vi "find.vi"() -> ()   [LabVIEW 2009]
uses:
  newCore/Variables/GlobalConAxisPI.vi
  newCore/Camera/lib/System Files/user.lib/atmcd32d.llb/Shutter_type typedef.ctl
  newCore/Camera/lib/System Files/user.lib/atmcd32d.llb/Shutter_mode typedef.ctl
  newCore/Camera/vi/GlobalSetGetConfigureCamera.vi
  newCore/Camera/vi/ccdChipPixels.vi
  <vilib>/vision/Image Controls.llb/IMAQ Rounding Mode.ctl
  newCore/Variables/patternImg.vi
  <vilib>/vision/Pattern Matching.llb/IMAQ Match Range Setting.ctl
  <vilib>/vision/Pattern Matching.llb/IMAQ Curve Parameters.ctl
panel:
  in  "Tab Control":T1(tab)
  out "Histogram":i32[][](graph)
  out "Trace":i32[][](graph)
  out "Point":dbl[][](graph)
  out "Image Out":T2(plugin-control)
  out "Image Number":u32
  out "acquired FPS":dbl
  out "Image":i32[][](graph)
  out "AM image":T2(plugin-control)
  out "Number of Particles":i32
  out "Image 2":dbl[][](graph)
  out "concatenated string":string
  out "Task":T3(ring)
  in  "PI SystemNumber":i32
  in  "WS File Tree":string(tree)
  out "Active pt3":path
  out "Workspace":path
  out "Stop Measurement":bool
  out "Buffer Overrun":bool
  out "Running":bool
  out "Global Stop":bool
  out "x-position":dbl format="%.3f"
  out "y-position":dbl format="%.3f"
  out "z-position":dbl format="%.3f"
  out "Auto Meas Progress":i32(slide) caption="Point 34 / 34"
  out "NxtAutMesPoint":i32
  out "Auto Measure Points":i32
  out "subarray":dbl[](array[numeric])
  out "Pattern":dbl[][](array[numeric])
  in  "Remove Outliers":i32
  in  "Filter":bool
  in  "Exclude / Include X":bool
  in  "X Start 2":dbl
  in  "X End 2":dbl
  in  "Y Start 2":dbl
  in  "Y End 2":dbl
  in  "Exclude / Include Y":bool
  in  "Measurement Parameter 1":T4 items=["Center of Mass X", "Center of Mass Y", "First Pixel X", "First Pixel Y", "Bounding Rect Left", "Bounding Rect Top", "Bounding Rect Right", "Bounding Rect Bottom", "Max Feret Diameter Start X", "Max Feret Diameter Start Y", "Max Feret Diameter End X", "Max Feret Diameter End Y", "Max Horiz. Segment Length Left", "Max Horiz. Segment Length Right", "Max Horiz. Segment Length Row", "-", "Bounding Rect Width", "Bounding Rect Height", "Bounding Rect Diagonal", "Perimeter", "Convex Hull Perimeter", "Holes' Perimeter", "Max Feret Diameter", "Equivalent Ellipse Major Axis", "Equivalent Ellipse Minor Axis", "Equivalent Ellipse Minor Axis (Feret)", "Equivalent Rect Long Side", "Equivalent Rect Short Side", "Equivalent Rect Diagonal", "Equivalent Rect Short Side (Feret)", "Average Horiz. Segment Length", "Average Vert. Segment Length", "Hydraulic Radius", "Waddel Disk Diameter", "-", "Area", "Holes' Area", "Particle & Holes' Area", "Convex Hull Area", "Image Area", "-", "Number of Holes", "Number of Horiz. Segments", "Number of Vert. Segments", "-", "Orientation", "Max Feret Diameter Orientation", "-", "% Area/Image Area", "% Area/(Particle & Holes' Area)", "Ratio of Equivalent Ellipse Axes", "Ratio of Equivalent Rect Sides", "-", "Elongation Factor", "Compactness Factor", "Heywood Circularity Factor", "Type Factor", "-", "Sum X", "Sum Y", "Sum XX", "Sum XY", "Sum YY", "Sum XXX", "Sum XXY", "Sum XYY", "Sum YYY", "-", "Moment of Inertia XX", "Moment of Inertia XY", "Moment of Inertia YY", "Moment of Inertia XXX", "Moment of Inertia XXY", "Moment of Inertia XYY", "Moment of Inertia YYY", "Norm. Moment of Inertia XX", "Norm. Moment of Inertia XY", "Norm. Moment of Inertia YY", "Norm. Moment of Inertia XXX", "Norm. Moment of Inertia XXY", "Norm. Moment of Inertia XYY", "Norm. Moment of Inertia YYY", "Hu Moment 1", "Hu Moment 2", "Hu Moment 3", "Hu Moment 4", "Hu Moment 5", "Hu Moment 6", "Hu Moment 7"]
  in  "Range Lower Value Par 1":dbl
  in  "Range Upper Value  Par 1":dbl
  in  "Ex/In Par 1":bool
  in  "Measurement Parameter 2":T4 items=["Center of Mass X", "Center of Mass Y", "First Pixel X", "First Pixel Y", "Bounding Rect Left", "Bounding Rect Top", "Bounding Rect Right", "Bounding Rect Bottom", "Max Feret Diameter Start X", "Max Feret Diameter Start Y", "Max Feret Diameter End X", "Max Feret Diameter End Y", "Max Horiz. Segment Length Left", "Max Horiz. Segment Length Right", "Max Horiz. Segment Length Row", "-", "Bounding Rect Width", "Bounding Rect Height", "Bounding Rect Diagonal", "Perimeter", "Convex Hull Perimeter", "Holes' Perimeter", "Max Feret Diameter", "Equivalent Ellipse Major Axis", "Equivalent Ellipse Minor Axis", "Equivalent Ellipse Minor Axis (Feret)", "Equivalent Rect Long Side", "Equivalent Rect Short Side", "Equivalent Rect Diagonal", "Equivalent Rect Short Side (Feret)", "Average Horiz. Segment Length", "Average Vert. Segment Length", "Hydraulic Radius", "Waddel Disk Diameter", "-", "Area", "Holes' Area", "Particle & Holes' Area", "Convex Hull Area", "Image Area", "-", "Number of Holes", "Number of Horiz. Segments", "Number of Vert. Segments", "-", "Orientation", "Max Feret Diameter Orientation", "-", "% Area/Image Area", "% Area/(Particle & Holes' Area)", "Ratio of Equivalent Ellipse Axes", "Ratio of Equivalent Rect Sides", "-", "Elongation Factor", "Compactness Factor", "Heywood Circularity Factor", "Type Factor", "-", "Sum X", "Sum Y", "Sum XX", "Sum XY", "Sum YY", "Sum XXX", "Sum XXY", "Sum XYY", "Sum YYY", "-", "Moment of Inertia XX", "Moment of Inertia XY", "Moment of Inertia YY", "Moment of Inertia XXX", "Moment of Inertia XXY", "Moment of Inertia XYY", "Moment of Inertia YYY", "Norm. Moment of Inertia XX", "Norm. Moment of Inertia XY", "Norm. Moment of Inertia YY", "Norm. Moment of Inertia XXX", "Norm. Moment of Inertia XXY", "Norm. Moment of Inertia XYY", "Norm. Moment of Inertia YYY", "Hu Moment 1", "Hu Moment 2", "Hu Moment 3", "Hu Moment 4", "Hu Moment 5", "Hu Moment 6", "Hu Moment 7"]
  in  "Range Lower Value Par 2":dbl
  in  "Range Upper Value Par 2":dbl
  in  "Ex/In Par 2":bool
  in  "Settings (GeometricMatching)":T7 {"Curve Parameters"."Extraction Mode" items=["Normal", "Uniform Regions"]; "Curve Parameters"."Edge Filter Size" items=["Fine", "Normal", "Contour Tracing"]; "Curve Parameters"."Max Endpoint Gap" min=0; "Curve Parameters"."Col Search Step Size" min=1 max=255 step=1; "Curve Parameters"."Row Search Step Size" min=1 max=255 step=1; "Curve Parameters"."Min Length" min=0; "Curve Parameters"."Edge Threshold" min=1 max=350 step=1; "Range Settings"."Max" format="%.2f"; "Range Settings"."Min" format="%.2f"; "Range Settings"."Match Constraints" items=["Rotation Angle (degrees)", "Scale Factor (%)", "Occlusion (%)"]; "Adv. Geometric Match Options 2"."Setup Data Item" items=["Curve Extraction Mode", "Curve Edge Threshold", "Curve Edge Filter Size", "Min Curve Length", "Curve Row Search Step Size", "Curve Col Search Step Size", "Curve Max Endpoint Gap", "Extract Closed Curves", "Enable Subpixel Curve Extraction", "Enable Correlation Score", "Enable Subpixel Accuracy", "Subpixel Iterations", "Subpixel Tolerance", "Initial Match List Length", "Enable Target Template Curve Score", "Min Match Separation Distance", "Min Match Separation Angle", "Min Match Separation Scale", "Max Match Overlap", "Enable Coarse Result", "Enable Calibration Support", "Enable Contrast Reversal", "Search Strategy", "Refinement Match Factor", "Subpixel Match Factor"]}
  in  "Square/Hexa":bool
  in  "Connectivity 4/8":bool
  in  "Manual":bool
  in  "Mode":enum16{"Gauss", "Radial", "Azimuthal"}(ring)
  in  "Focuswidth":dbl
  in  "Detection Modus":u16(ring) items=["Pattern", "Heuristic"]
  in  "NA":dbl
  in  "Measurement Time":i32 min=10 format="%.0d s"
  out "Counts":u32[](array[numeric])
  in  "Adjustment":bool
  in  "Autopoint-Autofocus Z":bool
  in  "Auto Measurement Time (ms)":i32 caption="Measurement Time (s)" min=10
  in  "Auto Defocussed Cam":bool
  in  "Point Defocussed Cam":bool
  in  "X-Position":dbl caption="X" min=0.0 max=200.0 step=0.1 format="%1.3f um"
  in  "Y-Position":dbl caption="Y" min=0.0 max=200.0 step=0.1 format="%1.3f um"
  in  "Z-Position":dbl caption="Z" min=0.0 max=200.0 step=0.1 format="%1.3f um"
  in  "Picture size":dbl min=0.1 max=200.0 format="%1.1f um"
  in  "Picture size 2":dbl min=0.1 max=200.0 format="%1.1f um"
  in  "Pixel time":dbl min=0.1 max=100.0 step=0.1 format="%.1f ms"
  in  "Resolution":dbl min=0.01 max=10.0 step=0.01 format="%.2f µm"
  in  "Laser  Profile":string
  in  "Save Files":bool
  in  "Axis":enum32{"x-y", "x-z", "y-x", "y-z", "z-x", "z-y"}(ring)
  out "Last Image File No":i32
  in  "CFD Settings":T8
  out "Measure. time":dbl format="%7.1f s"
  in  "Laser pulse duration":i32[](array[numeric]) min=2 max=100000 step=1 format="%d µs"
  # "Range"
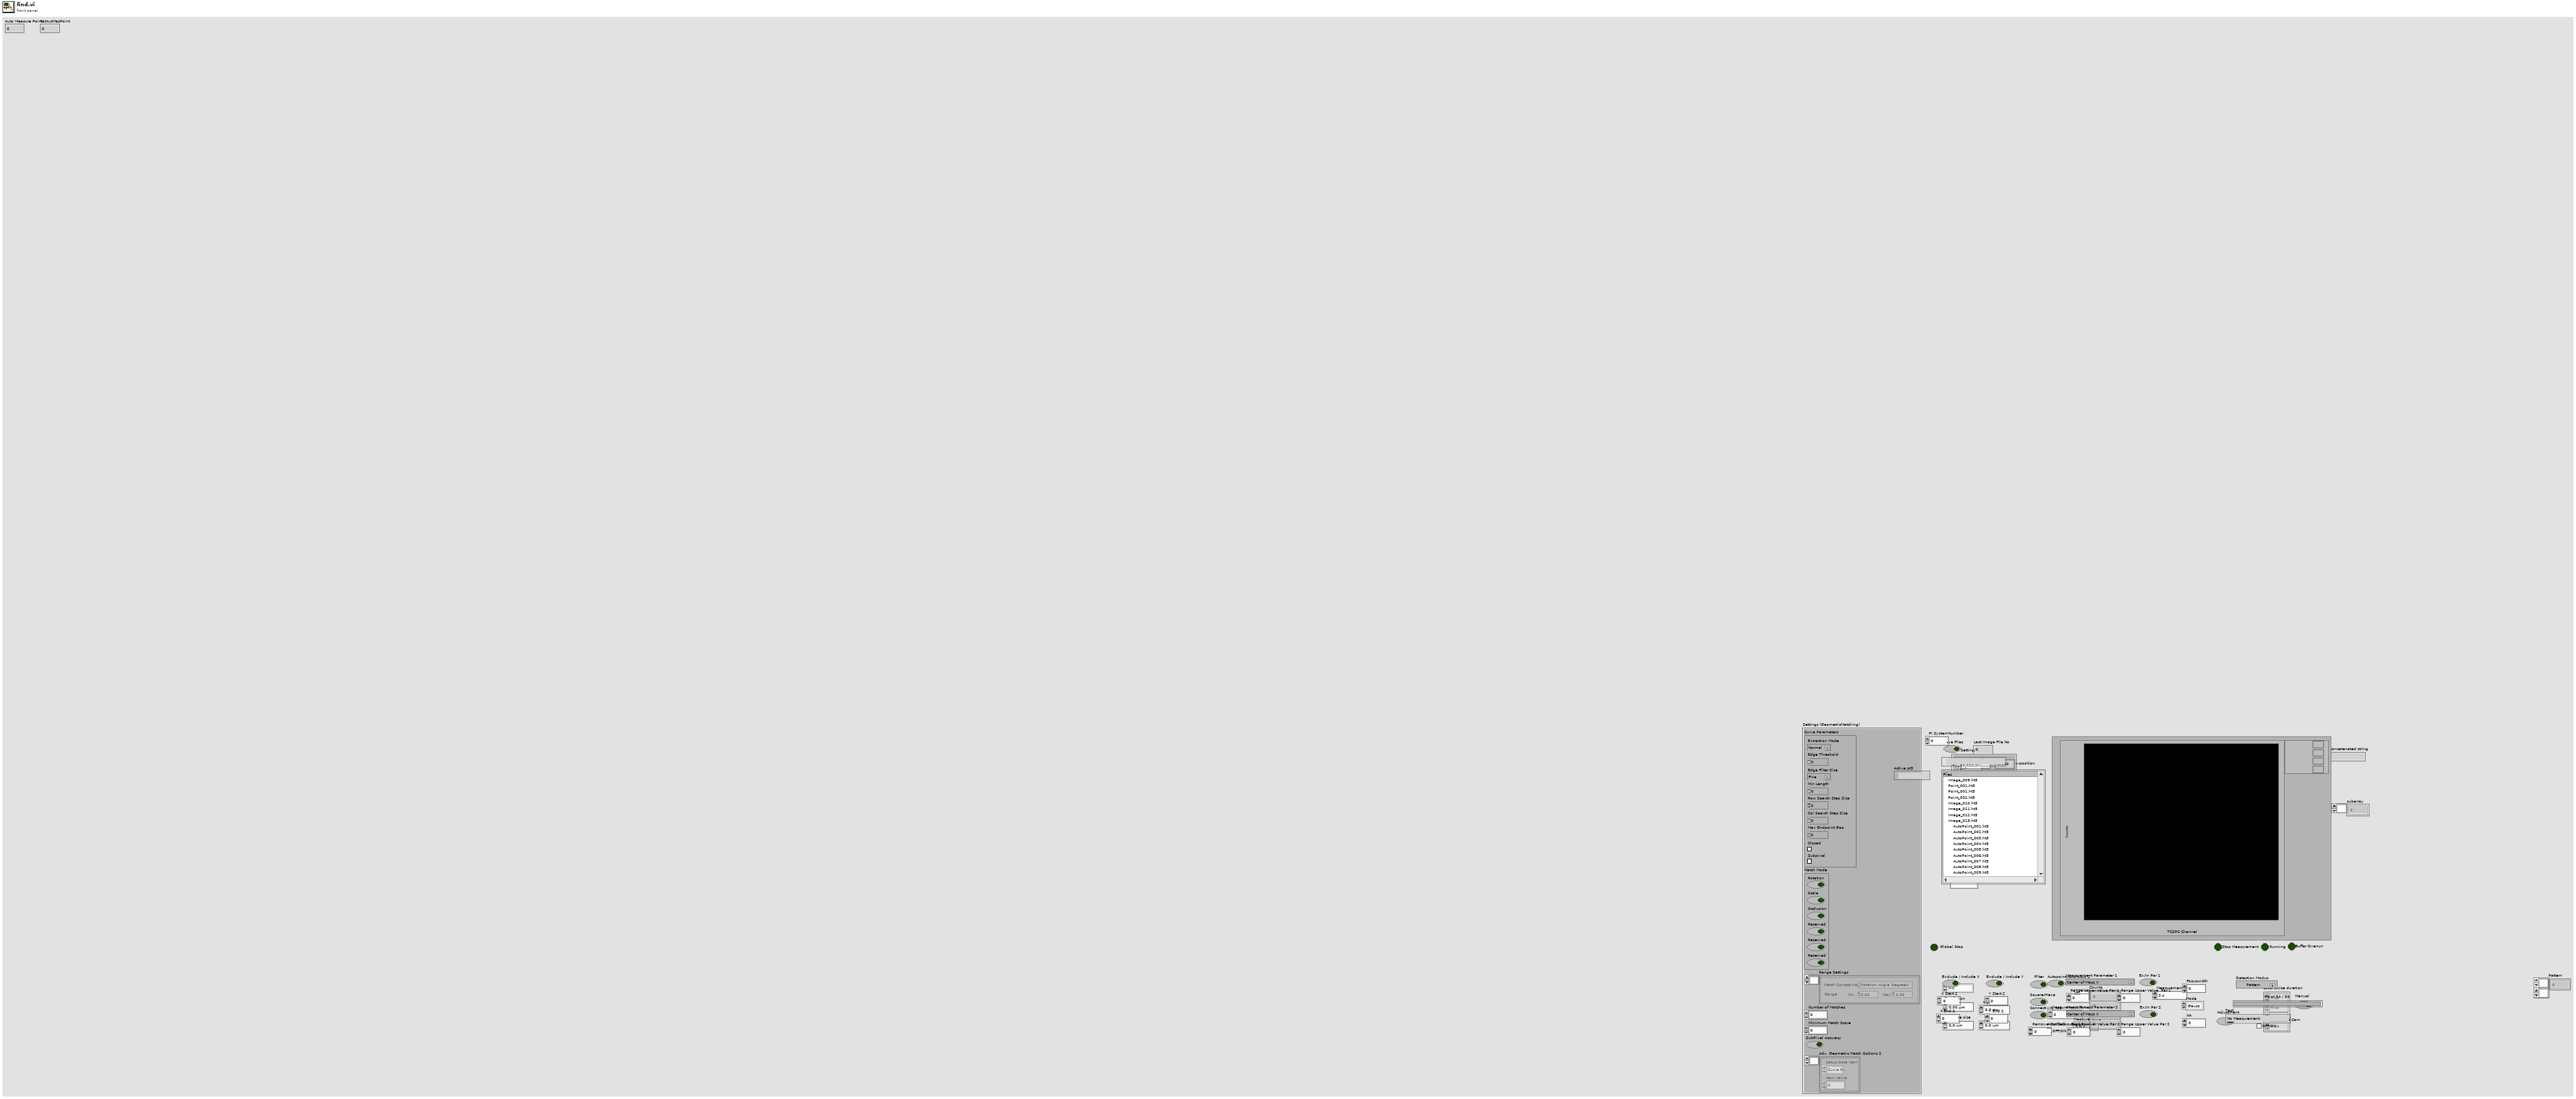
[diagram p1: front panel]
types:
  T1 = enum32{"TCSPC Histogram", "Trace", "CCD", "Backreflection", "Image", "AutoMesaurement"}
  T2 = typedef "IMAQ Image.ctl" = refnum<image>
  T3 = enum16{"No Measurement", "Aquire Image", "Point Measurement", "Multi Measurement", "Save Color Image", "Find Single Mol.", "Auto Measurement Control", "Auto Point", "Aquire Line Scan", "Grid Measurement", "Trapping", "Move Scanner"}
  T4 = typedef "Particle Parameters" = i32
  T5 = typedef "IMAQ Curve Parameters.ctl" = cluster{"Extraction Mode":u32, "Edge Threshold":i32, "Edge Filter Size":u32, "Min Length":i32, "Row Search Step Size":i32, "Col Search Step Size":i32, "Max Endpoint Gap":i32, "Closed":bool, "Subpixel":bool}
  T6 = typedef "IMAQ Match Range Setting.ctl" = cluster{"Match Constraints":u32, "Min":dbl, "Max":dbl}
  T7 = cluster{"Curve Parameters":T5, "Match Mode":cluster{"Rotation":bool, "Scale":bool, "Occlusion":bool, "Reserved":bool, "Reserved":bool, "Reserved":bool}, "Range Settings":T6[], "Number of Matches":i32, "Minimum Match Score":sgl, "SubPixel Accuracy":bool, "Adv. Geometric Match Options 2":cluster{"Setup Data Item":u16, "Item Value":dbl}[]}
  T8 = cluster{"Sync Level":i32, "Sync ZeroX":i32, "Sync Offset":i32, "Chan Settings":cluster{"CHx Level":i32, "CHx ZeroX":i32, "CHx Offset":i32}[]}
  T9 = enum16{"No Measurement", "Aquire Image", "Point Measurement", "Multi Measurement", "Save Color Image", "Find Single Mol.", "Auto Measurement Control", "Auto Point", "Aquire Line Scan", "Grid Measurement"}
  T10 = enum16{"none", "fast axis", "slow axis", "both axis", ""}
  T11 = enum16{"none", "fast axis", "slow axis", "both", ""}
  T12 = enum16{"target position", "relative position", "actual position", "position error"}
  T13 = enum16{"not a pt3 File", "Image File", "Point Measurement", "Auto Point"}
  T14 = enum16{"unknown", "pt3 File", "png Image", "bmp Image"}
  T15 = typedef "Shutter_mode typedef.ctl" = enum16{"Auto", "Open", "Close"}
  T16 = typedef "Shutter_type typedef.ctl" = enum16{"TTL Low", "TTL High"}
  T17 = enum16{"No Measurement", "Aquire Image", "Point Measurement", "Multi Measurement", "Save Color Image", "Find Single Mol.", "Auto Measurement Control", "Auto Point"}
  T18 = typedef "IMAQ Rounding Mode.ctl" = enum16{"Optimize", "Truncate"}
  T19 = cluster{"Measurement Parameter":T4, "Range Lower Value":dbl, "Range Upper Value":dbl, "Range":bool, "Measurement Type":bool}[]
  T20 = enum16{"not a pt3 File", "Image File", "Point Measurement", "Auto Point", "Line Scan"}
  T21 = cluster{"Comment":string, "Binning":i32, "Offset":i32, "AcquisitionTime (ms)":i32, "HardwareSerial":i32, "SyncDivider":i32, "Resolution (ps)":dbl, "CFD Settings":cluster{"Sync Level":i32, "Sync ZeroX":i32, "Sync Offset":i32, "Chan Settings":cluster{"CHx Level":i32, "CHx ZeroX":i32, "CHx Offset":i32}[]}, "ModuleInfo":cluster{"modelcode":i32, "versioncode":i32}[], "BaseResolution (ps)":dbl, "RefClockSource":i32, "ChanInfo":cluster{"CHx Level":i32, "CHx ZeroX":i32, "CHx Offset":i32, "CHx modidx":i32}[], "SyncRate":i32, "InputsEnabled":i64}
  T22 = cluster{"Dimensions":i32, "Time Per Pixel [ms]":dbl, "Acceleration":i32, "Pattern":i32, "X0":sgl, "Y0":sgl, "Z0":dbl, "PixX":i32, "PixY":i32, "PixResol":sgl, "TStartTo":sgl, "TStoptTo":sgl, "TStartFro":sgl, "TStopFro":sgl}
  T23 = cluster{"InpRateFilePos":i64, "StopAfterFilePos":i64}
  T24 = cluster{"X-Position":dbl, "Y-Position":dbl, "Z-Position":dbl}
  T25 = cluster{"File No":i32, "File Path":path, "Parent File":i32, "File Type":enum16{"unknown", "pt3 File", "png Image", "bmp Image"}, "Measurement Type":enum16{"not a pt3 File", "Image File", "Point Measurement", "Auto Point", "Line Scan", "Grid Scan"}, "Upper Left":cluster{"x-Position":dbl, "y-Position":dbl, "z-Position":dbl}, "Pixels":i32[], "Scan Axis":enum32{"x-y", "x-z", "y-z"}, "Resolution":dbl, "PixelTime":dbl}
  T26 = enum16{"not a pt3 File", "Image File", "Point Measurement", "Auto Point", "Line Scan", "Grid Scan"}
  T27 = cluster{"Ident":string, "Format Version":string, "Creator Name":string, "Creator Version":string, "File Time":string, "Comment":string, "Laser":i32, "Binning":i32, "Offset":i32, "AcquisitionTime (ms)":i32, "HardwareSerial":i32, "SyncDivider":i32, "Resolution (ps)":dbl, "Rates":dbl[], "SyncRate":dbl, "CFD Settings":cluster{"Sync Level":i32, "Sync ZeroX":i32, "Sync Offset":i32, "Chan Settings":cluster{"CHx Level":i32, "CHx ZeroX":i32, "CHx Offset":i32}[]}}
  T28 = cluster{"x-Position":dbl, "y-Position":dbl, "z-Position":dbl}
  T29 = typedef "Image Type" = u32
  T30 = cluster{"MesaurementSelection[0]":cluster{"Measurement Parameter":T4, "Range Lower Value":dbl, "Range Upper Value":dbl, "Range":bool, "Measurement Type":bool}, "MesaurementSelection[1]":cluster{"Measurement Parameter":T4, "Range Lower Value":dbl, "Range Upper Value":dbl, "Range":bool, "Measurement Type":bool}, "MesaurementSelection[2]":cluster{"Measurement Parameter":T4, "Range Lower Value":dbl, "Range Upper Value":dbl, "Range":bool, "Measurement Type":bool}, "MesaurementSelection[3]":cluster{"Measurement Parameter":T4, "Range Lower Value":dbl, "Range Upper Value":dbl, "Range":bool, "Measurement Type":bool}, "MesaurementSelection[4]":cluster{"Measurement Parameter":T4, "Range Lower Value":dbl, "Range Upper Value":dbl, "Range":bool, "Measurement Type":bool}, "MesaurementSelection[5]":cluster{"Measurement Parameter":T4, "Range Lower Value":dbl, "Range Upper Value":dbl, "Range":bool, "Measurement Type":bool}, "MesaurementSelection[6]":cluster{"Measurement Parameter":T4, "Range Lower Value":dbl, "Range Upper Value":dbl, "Range":bool, "Measurement Type":bool}, "MesaurementSelection[7]":cluster{"Measurement Parameter":T4, "Range Lower Value":dbl, "Range Upper Value":dbl, "Range":bool, "Measurement Type":bool}, "MesaurementSelection[8]":cluster{"Measurement Parameter":T4, "Range Lower Value":dbl, "Range Upper Value":dbl, "Range":bool, "Measurement Type":bool}}
  T31 = cluster{"Measurement Parameter":T4, "Range Lower Value":dbl, "Range Upper Value":dbl, "Range":bool, "Measurement Type":bool}
  T32 = typedef "IMAQ Point" = cluster{"X":sgl, "Y":sgl}
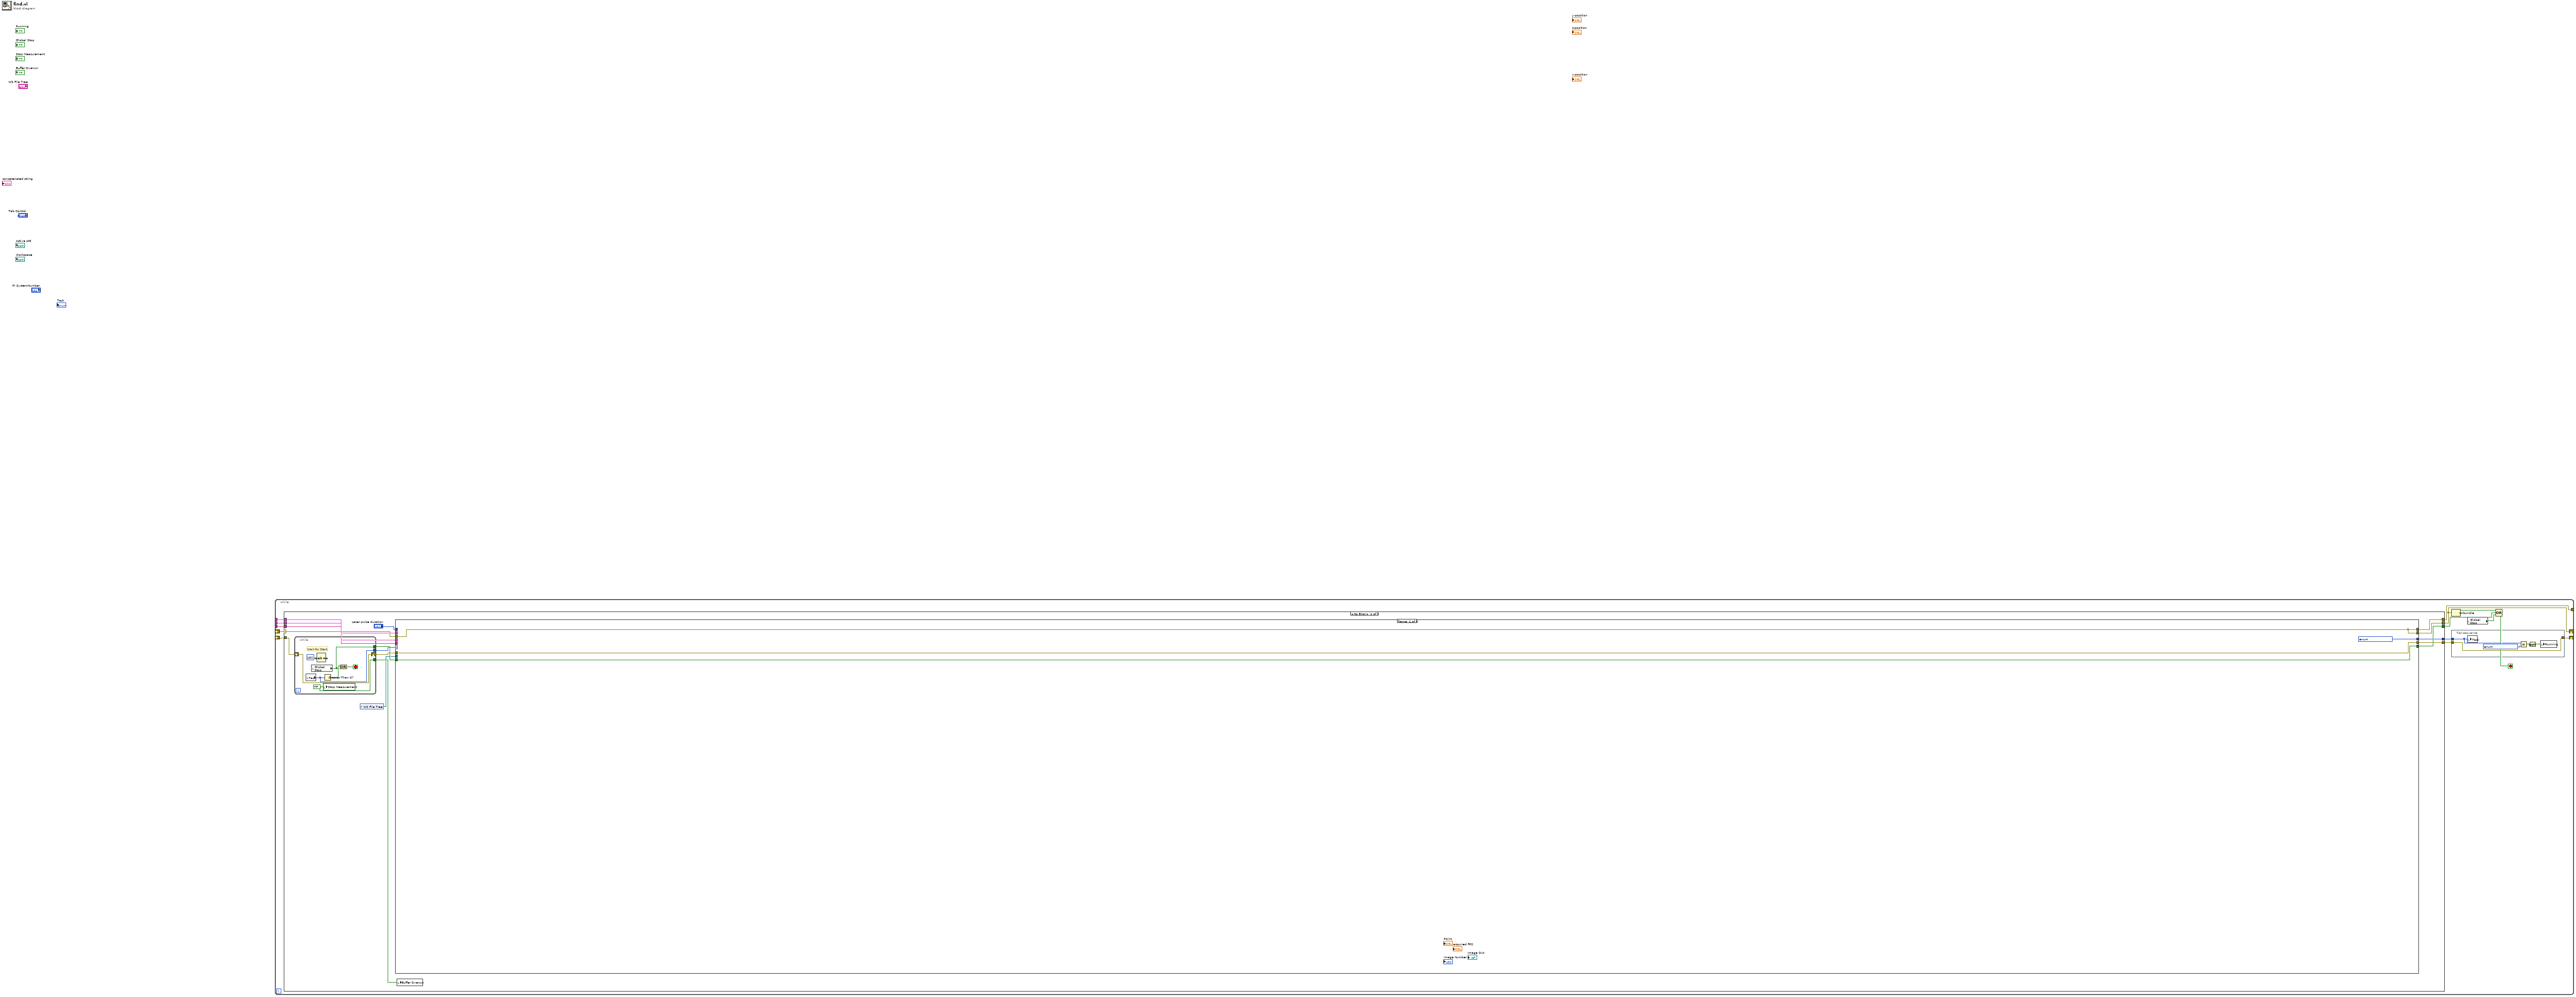
[diagram p0: block diagram]
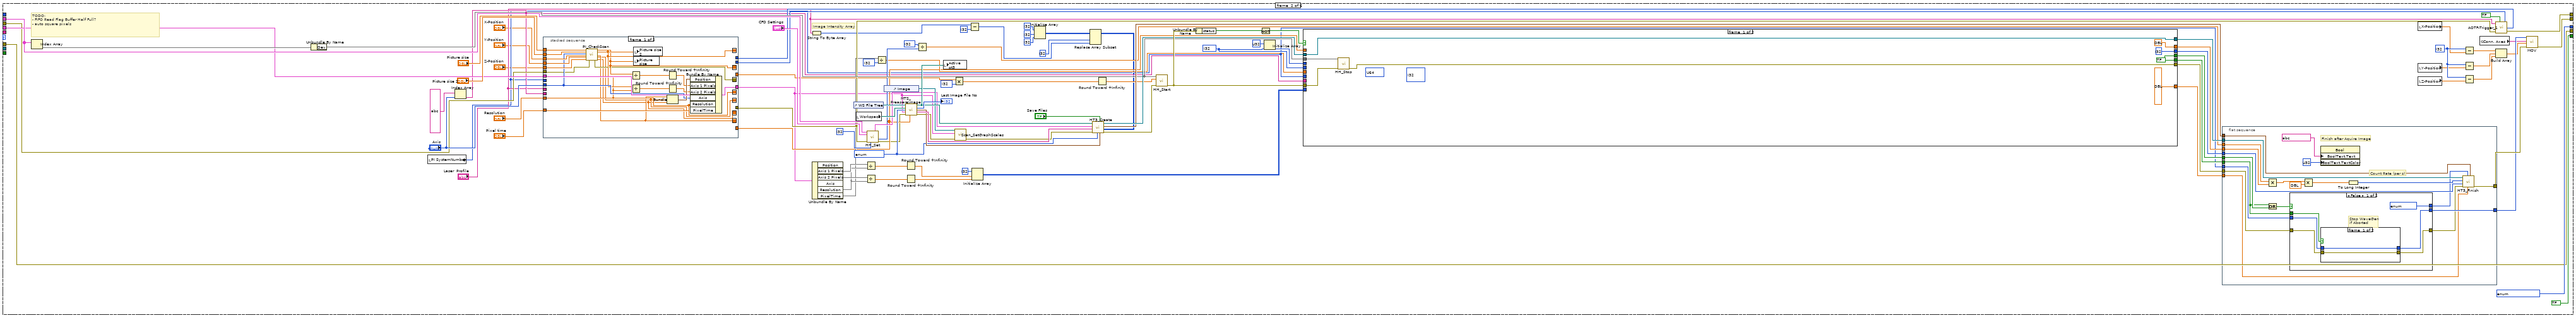
[diagram p2: hidden frame]
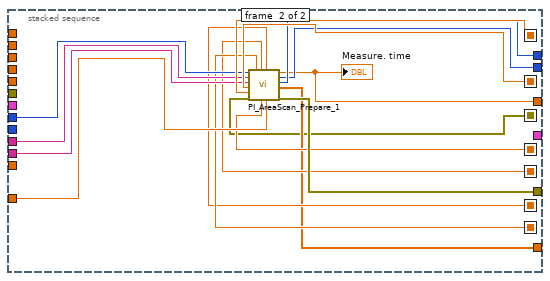
[diagram p3: hidden frame]
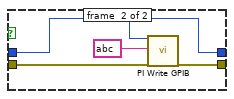
[diagram p4: hidden frame]
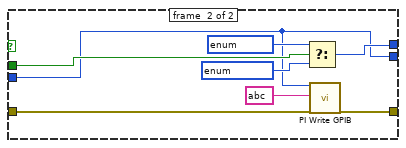
[diagram p5: hidden frame]
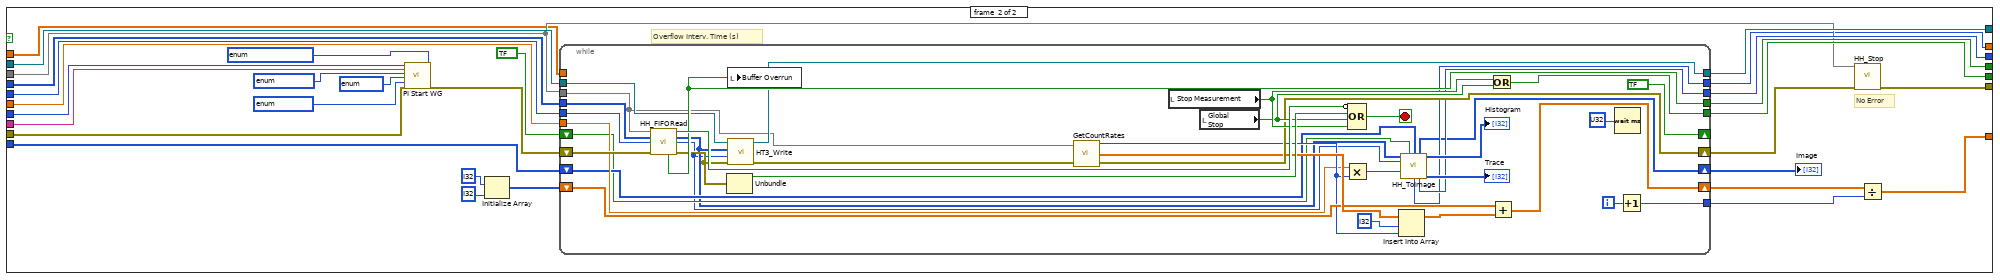
[diagram p6: hidden frame]
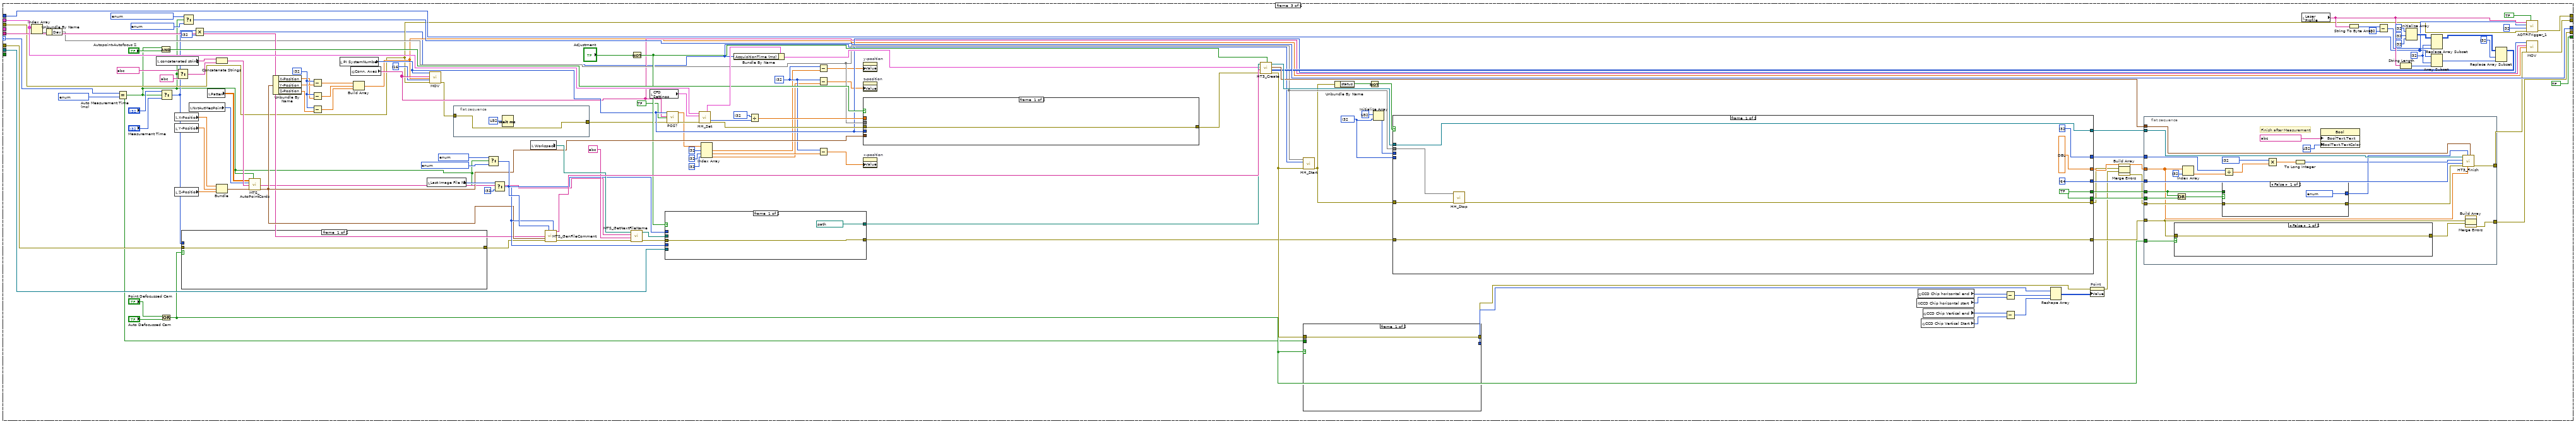
[diagram p7: hidden frame]
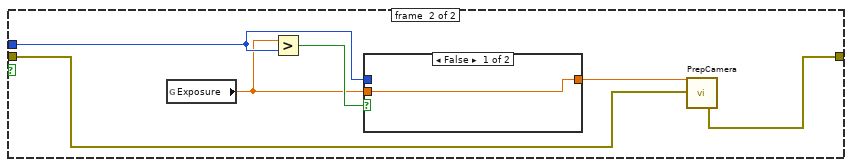
[diagram p8: hidden frame]
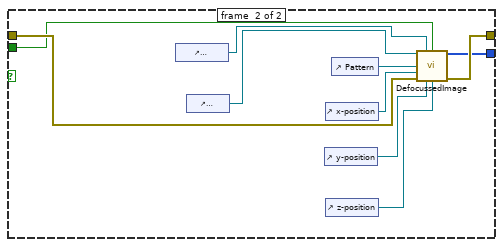
[diagram p10: hidden frame]
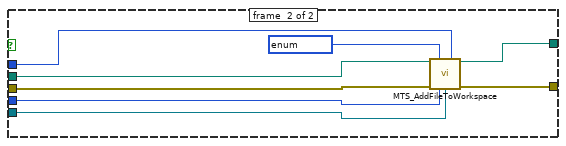
[diagram p11: hidden frame]
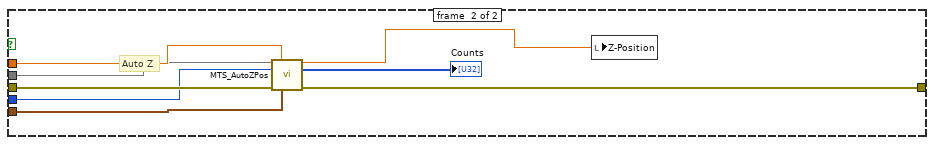
[diagram p12: hidden frame]
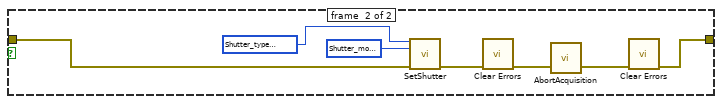
[diagram p13: hidden frame]
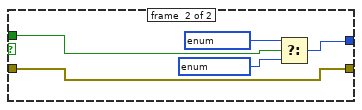
[diagram p14: hidden frame]
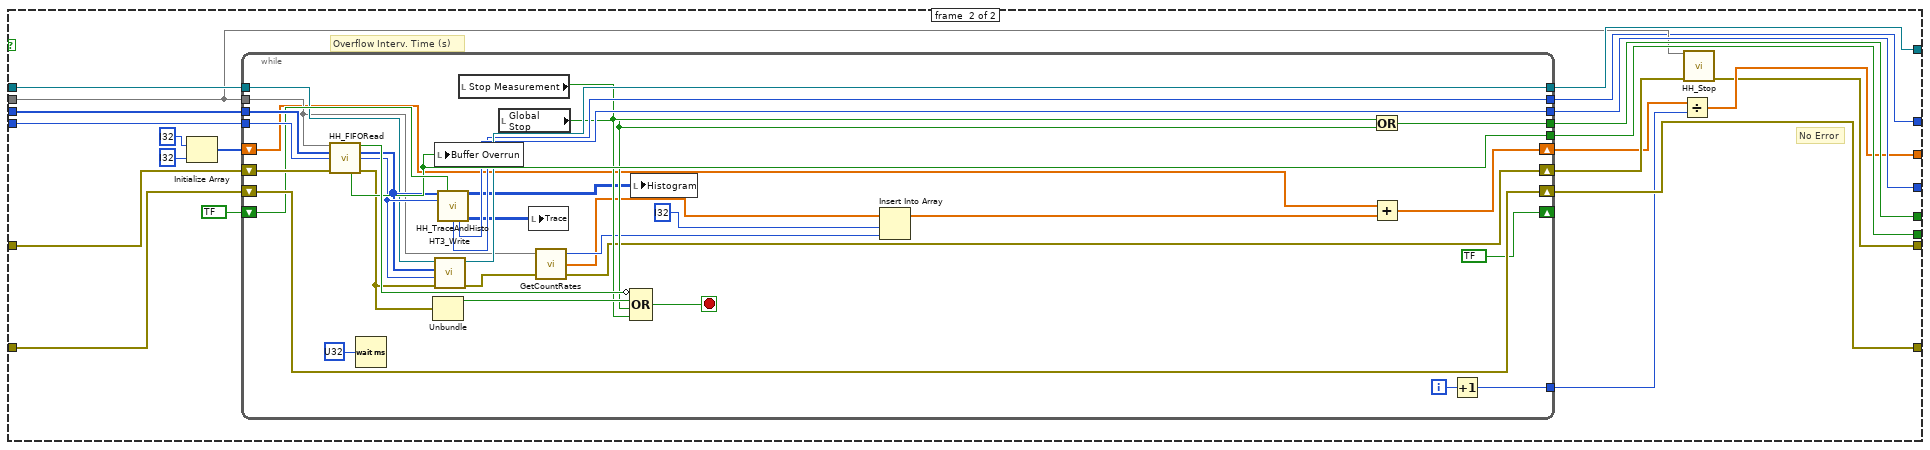
[diagram p15: hidden frame]
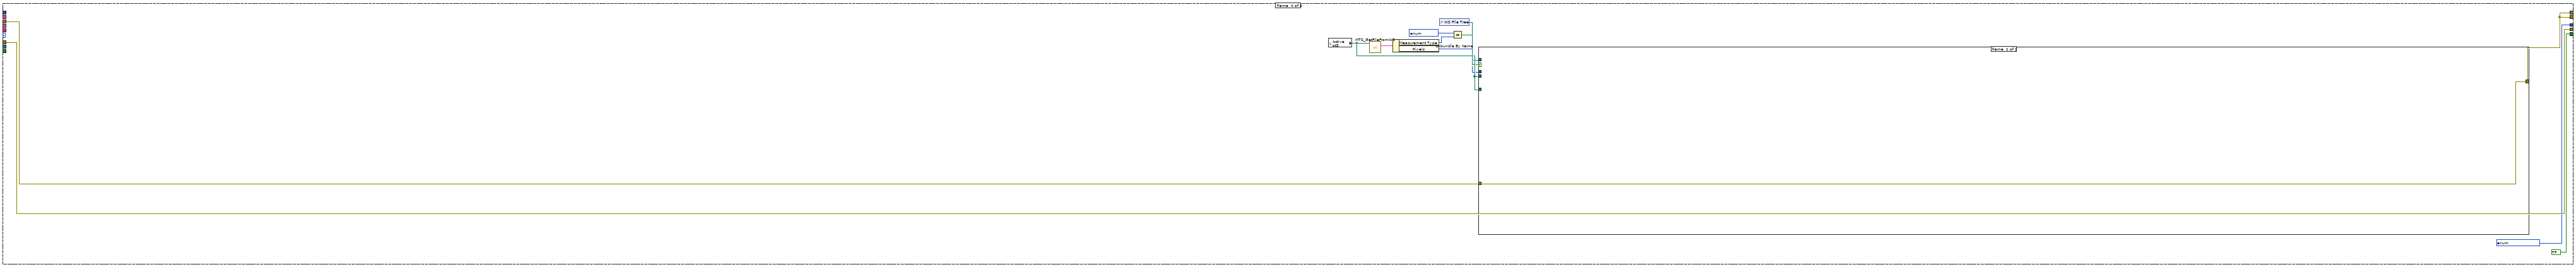
[diagram p16: hidden frame]
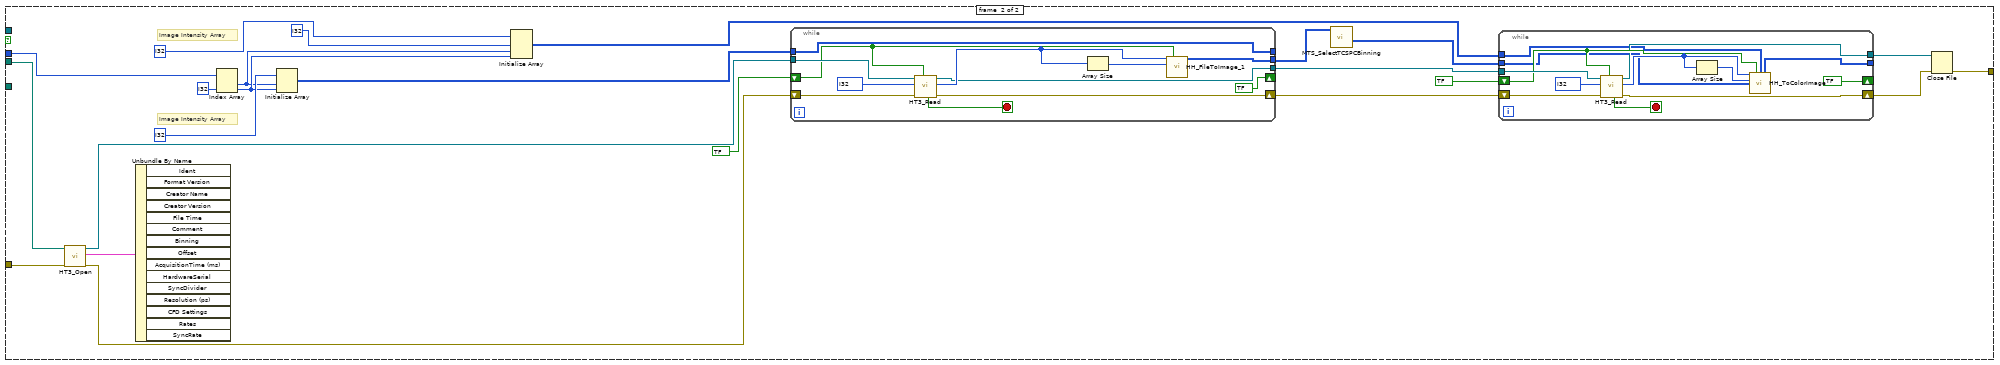
[diagram p17: hidden frame]
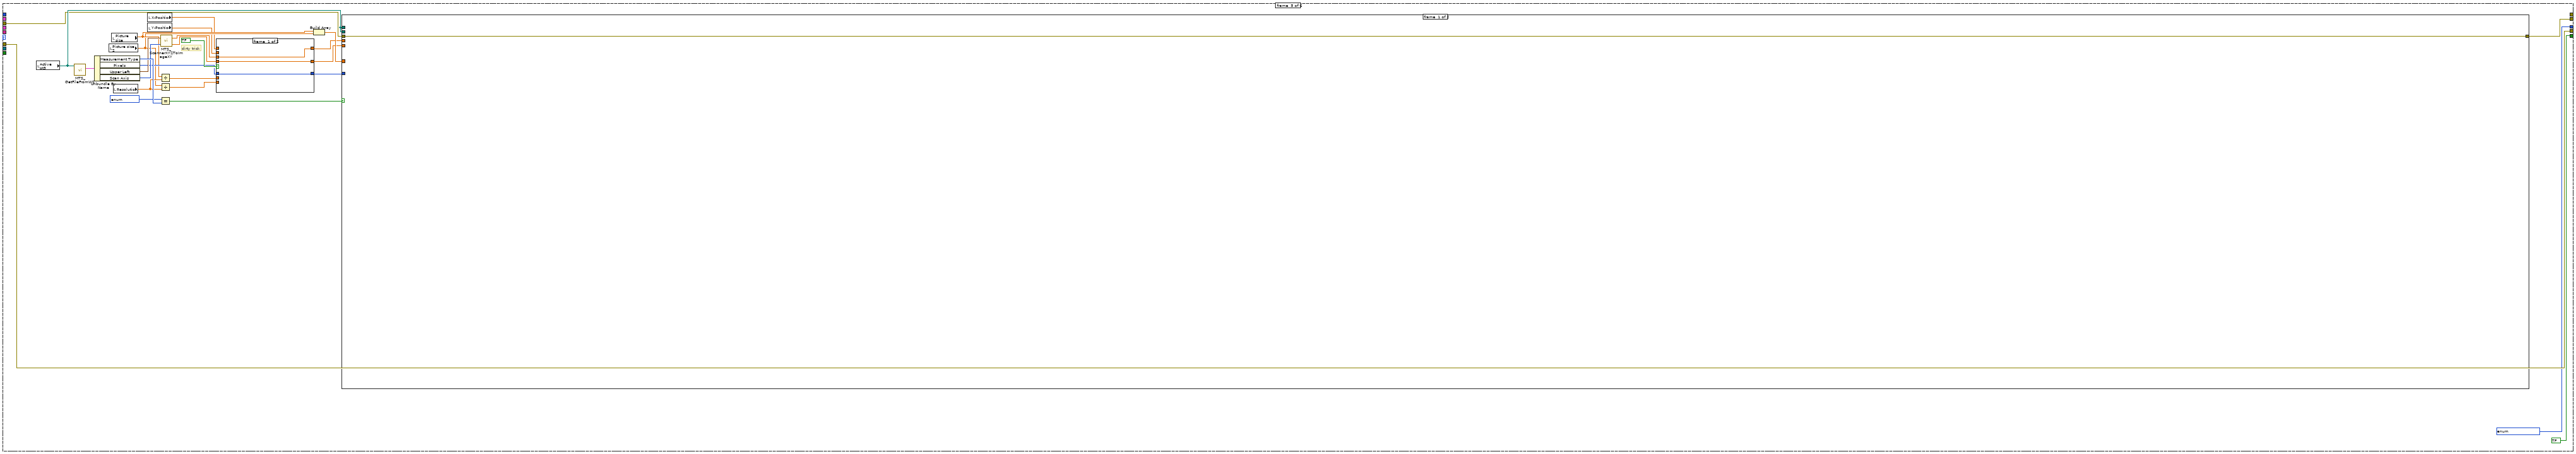
[diagram p18: hidden frame]
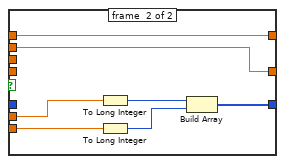
[diagram p19: hidden frame]
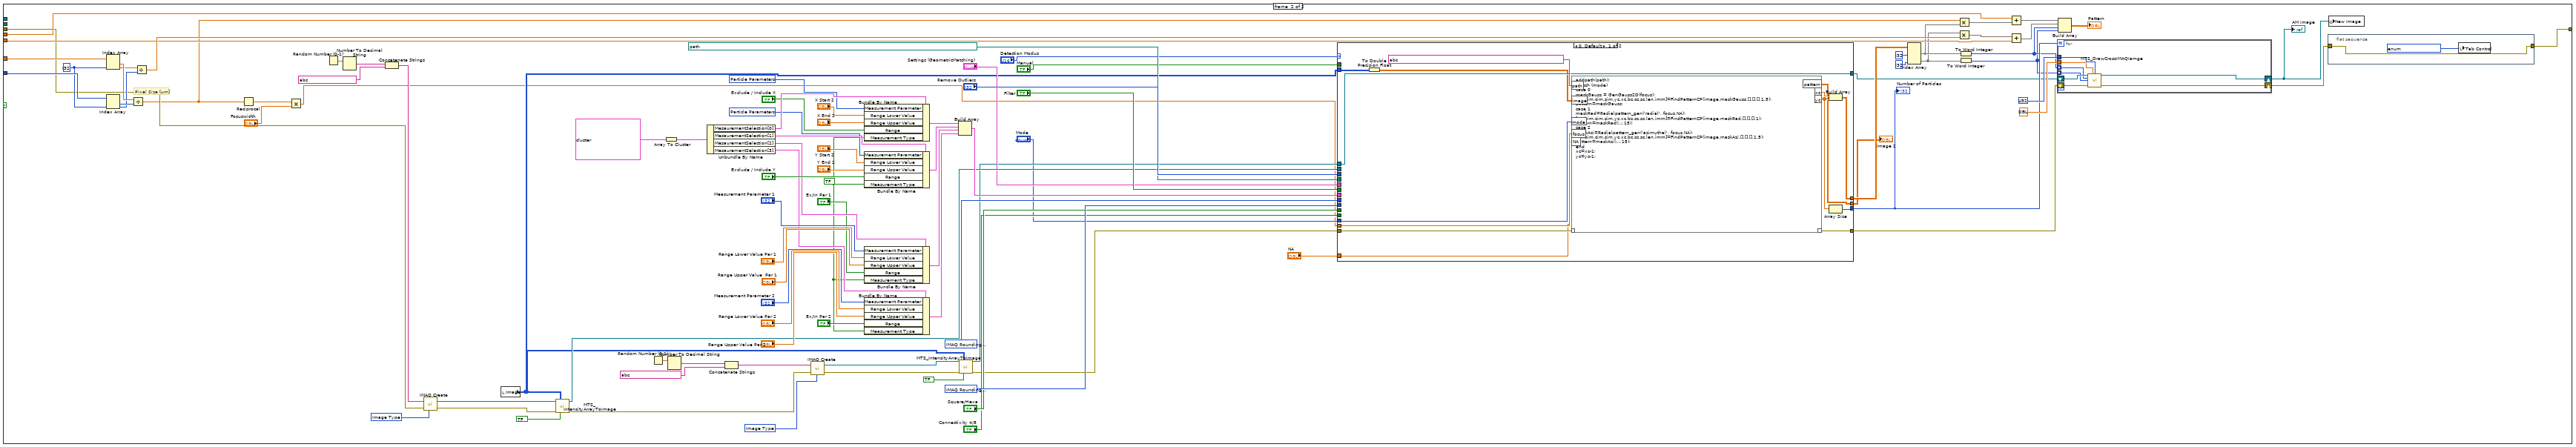
[diagram p20: hidden frame]
diagram:
  n1 = while {
    shift-right: [w7] -> _
    shift-left: _ -> [w4]
    shift-right: [w9] -> _
    shift-left: _ -> [w14]
    tunnel: _ -> [w8]
    tunnel: _ -> [w3]
    tunnel: [w2] -> _
    tunnel: _ -> [w1]
    stop <- w12 stop-if-true
    n2 = case shown="No Error" w4 {
      selector: w4 -> [w20 w892]
      tunnel: w14 -> [w30 w894]
      tunnel: [w29 bool ? ("Global Stop")] -> w11
      tunnel: [w25 w894] -> w10
      tunnel: w8 -> [w24 _]
      tunnel: [w23 w892] -> w7
      tunnel: [w21 T9 ? ("Do Measurement")] -> w5
      tunnel: w3 -> [w18 _]
      tunnel: [w17 w892] -> w2
      tunnel: w1 -> [w15 _]
      frame #0 {
        n3 = while {
          shift-right: [w890] -> w26
          shift-left: w30 -> [w890]
          tunnel: [w885] -> w28
          tunnel: [w887] -> w27
          tunnel: [w886] -> w22
          stop <- w891 stop-if-true
          w886 = bool ? ("FiFo Overrun")
          # "Wait for Start"
          n4 = local read "Task"() -> (w885:T3)
          n5 = local read "Global Stop"() -> (w887:bool)
          n6 = Wait (ms)(milliseconds to wait=u32 ?) -> ()  [unwired: 1 out]
          n7 = Greater Than 0?(x=w885) -> (x > 0?=w889:bool)
          n8 = local write "Stop Measurement"(w886) -> ()
          n9 = Or(x=w889, y=w887) -> (x .or. y?=w891:bool)
        }
        n10 = control-ref of="WS File Tree"() -> (w19:refnum<vi>)
        n11 = case shown="\"Find Single Mol.\"" w28 {
          selector: w28 -> [_ _ w397 _ _ _]
          tunnel: w20 -> [w31 w79 w305 w580 w649 w848]
          tunnel: [w31 w49 w353 w569 w647 w848] -> w23
          tunnel: [w32 bool ? ("Global Stop") bool ? ("Global Stop") bool ? ("Global Stop") bool ? ("Global Stop") bool ? ("Global Stop")] -> w29
          tunnel: w27 -> [w32 _ _ _ _ _]
          tunnel: w26 -> [w34 w63 w304 w579 w648 w849]
          tunnel: [w34 w63 w418 w579 w648 w847] -> w25
          tunnel: w24 -> [_ w129 w355 _ _ _]
          tunnel: [T9 ? ("Do Measurement") T9 ? ("Do Measurement") w396 T9 ? ("Do Measurement") T17 ? ("Do Measurement") w846] -> w21
          tunnel: w19 -> [_ _ w386 _ _ _]
          tunnel: w18 -> [_ w107 _ _ _ _]
          tunnel: [w31 w81 w379 w569 _ _] -> w17
          tunnel: "Laser pulse duration" -> [_ _ w361 _ _ _]
          tunnel: w15 -> [_ _ w352 _ _ _]
          frame #0 {
          }
          frame #1 {
            w42 = i32 ?
            w73 = T20 ? ("Measurement Type")
            w110 = i32 ? ("dimension size")
            # "TODO:\n- FIFO Read Flag Buffer Half Full?\n- auto square pixels"
            # "Image Intensity Array"
            n12 = Index Array(array=w129) -> (element=w128)  [unwired: 1 in]
            n13 = Unbundle By Name(w128) -> ("Dev"=w101)
            n14 = local read "PI SystemNumber"() -> (w51:i32)
            n15 = Index Array(array=string[] ? ("Array"), index="Axis") -> (element=w56:string)
            n16 = stacked-sequence {
              seq-local: [w141 _] -> [_ w168]
              seq-local: [w140 _] -> [_ w169]
              seq-local: [w139 _] -> [_ w164]
              seq-local: [w135 _] -> [_ w162]
              seq-local: [w134 _] -> [_ w161]
              seq-local: [w133 _] -> [_ w160]
              seq-local: [w136 _] -> [_ w156]
              tunnel: "Picture size" -> [w154 _]
              tunnel: "Picture size 2" -> [w153 _]
              tunnel: w107 -> [w152 _]
              tunnel: "X-Position" -> [w151 _]
              tunnel: "Y-Position" -> [w150 _]
              tunnel: "Z-Position" -> [w149 _]
              tunnel: "Axis" -> [w143 _]
              tunnel: "Resolution" -> [w139 _]
              tunnel: [w142 _] -> w35
              tunnel: [_ w170] -> w80
              tunnel: w79 -> [w137 _]
              tunnel: w56 -> [_ w167]
              tunnel: "Laser  Profile" -> [_ w166]
              tunnel: "Pixel time" -> [w138 w165]
              tunnel: w51 -> [_ w163]
              tunnel: [_ w155] -> w76
              tunnel: [_ w159] -> w75
              tunnel: [_ w158] -> w74
              tunnel: [_ w157] -> w66
              frame #0 {
                n17 = call "PI_CheckScan.vi"("Picture size"=w154, "Picture size 2"=w153, "Axis"=w143, "x-Position"=w151, "y-Position"=w150, "z-Position"=w149, "error in (no error)"=w137) -> ("error out"=w136:errorcluster, "Picture size out"=w140:dbl, "Picture size out 2"=w141:dbl, "a0"=w135:dbl, "b0"=w134:dbl, "c0"=w133:dbl)  [unwired: 7 in]
                n18 = Divide(x=w140, y=w139) -> (x/y=w146:dbl)
                n19 = Divide(x=w141, y=w139) -> (x/y=w147:dbl)
                n20 = local write "Picture size 2"(w141) -> ()
                n21 = local write "Picture size"(w140) -> ()
                n22 = Round Toward +Infinity(x=w146) -> (ceil(x): smallest int >= x=w145:dbl)
                n23 = Round Toward +Infinity(x=w147) -> (ceil(x): smallest int >= x=w144:dbl)
                n24 = Bundle("a0"=w135, "b0"=w134, "c0"=w133) -> (w148:cluster{"a0":dbl, "b0":dbl, "c0":dbl})  [unwired: 1 in]
                n25 = Bundle By Name(cluster=w152, "Position"=w148, "Axis 1 Pixels"=w145, "Axis 2 Pixels"=w144, "Axis"=w143, "Resolution"=w139, "PixelTime"=w138) -> (w142:cluster{})
              }
              frame #1 {
                n26 = call "PI_AreaScan_Prepare_1.vi"("System"=w163, "Laser"=w166, "Axis"=w167, "da"=w169, "db"=w168, "error in (no error)"=w156, "a0"=w162, "b0"=w161, "Resolution"=w164, "c0"=w160, "Pixel time"=w165) -> ("Tacq"=w155:dbl, "lp"=w158:i32, "ap"=w159:i32, "Trigger"=w157:dbl[], "error out"=w170:errorcluster)  [unwired: 4 in]
                "Measure. time" <- w155
              }
            }
            n27 = String To Byte Array(string="Laser  Profile") -> (unsigned byte array=w58:u8[])
            n28 = Unbundle By Name(w35) -> ("Axis 1 Pixels"=w88, "Axis 2 Pixels"=w89, "Resolution"=w86, "PixelTime"=w70)  [unwired: 2 out]
            n29 = control-ref of="WS File Tree"() -> (w113:refnum<vi>)
            n30 = local read "Workspace"() -> (w118:path)
            n31 = Divide(x=w88, y=w86) -> (x/y=w97:dbl)
            n32 = Divide(x=w89, y=w86) -> (x/y=w99:dbl)
            n33 = call "HH_Set.vi"("Device List"=w129, "CFD Settings"="CFD Settings", "error in (no error)"=w80, "SyncDiv"=i32 ?) -> ("ht3 header out"=w93:T21, "Sync Rate"=w91:i32, "error out"=w65:errorcluster)  [unwired: 7 in, 2 out]
            n34 = Divide(x=w70, y=i32 ?) -> (x/y=w68:dbl)
            n35 = control-ref of="Image"() -> (w95:refnum<vi>)
            n36 = Round Toward +Infinity(x=w97) -> (ceil(x): smallest int >= x=w96:dbl)
            n37 = Round Toward +Infinity(x=w99) -> (ceil(x): smallest int >= x=w98:dbl)
            n38 = call "MTS_PreapareImage.vi"("WS File Tree"=w113, "Workspace"=w118, "Measurement Type"=w73, "Image Measurent Parameters"=w35, "error in"=w65, "Trigger"=w66) -> ("File Name (dup)"=w103:path, "File No"=→"Last Image File No":i32, "Image Header"=w105:T22, "Comment"=w106:string, "error out"=w64:errorcluster)  [unwired: 5 in]
            n39 = Divide(x=i32 ?, y=w91) -> (x/y=w72:dbl)
            n40 = local write "Active pt3"(w103) -> ()
            n41 = Multiply(x=w76, y=i32 ?) -> (x*y=w85:dbl)
            n42 = call "Scan_SetGraphScales.vi"("error in (no error)"=w64, "Image Measurent Parameters"=w35, "Image"=w95) -> ("error out"=w94:errorcluster)  [unwired: 8 in]
            n43 = Subtract(x=w58, y=i32 ?) -> (x-y=w57:i32[])
            n44 = Initialize Array(i32 ? ("element"), w96, w98) -> (w69:i32[][])
            n45 = Initialize Array(i32 ?, i32 ?, i32 ?) -> (w55:i32[][])
            n46 = Replace Array Subset(array=w55, new element=w57, index (col)=i32 ?) -> (w53:i32[][])  [unwired: 1 in]
            n47 = call "HT3_Create.vi"("Laser"=w53, "Image Header in"=w105, "Save pt3"="Save Files", "Measurement Type"=w73, "error in"=w94, "Comment"=w106, "ht3 Header in"=w93, "File Path"=w103) -> ("error out"=w119:errorcluster, "FileHeaderPos"=w109:T23, "refnum out"=w117:refnum<file>)  [unwired: 1 in]
            n48 = Round Toward +Infinity(x=w85) -> (ceil(x): smallest int >= x=w83:dbl)
            n49 = call "HH_Start.vi"("Device Index"=w101, "Acq. Time"=w83, "error in (no error)"=w119) -> ("error out"=w126:errorcluster)  [unwired: 11 in, 1 out]
            n50 = Unbundle By Name(w126) -> ("status"=w127:bool)
            n51 = Not(x=w127) -> (.not. x?=w125:bool)
            n52 = Initialize Array(u32 ?, w110) -> (w122:u32[])
            n53 = case shown="True" w125 {
              tunnel: [w218 w249] -> w124
              tunnel: w51 -> [_ w244]
              tunnel: w126 -> [w219 w245]
              tunnel: w101 -> [w217 w236]
              tunnel: w69 -> [_ w221]
              tunnel: w122 -> [_ w243]
              tunnel: w110 -> [_ w242]
              tunnel: [w216 w241] -> w121
              tunnel: [w216 w240] -> w120
              tunnel: w117 -> [w215 w239]
              tunnel: [w215 w238] -> w116
              tunnel: [i32 ? ("Num Records Total") w237] -> w115
              tunnel: [dbl ? w230] -> w114
              tunnel: w56 -> [_ w233]
              tunnel: [dbl[] ? w227] -> w71
              tunnel: w68 -> [_ w223]
              tunnel: w66 -> [_ w222]
              frame #0 {
                (unwired) i32[][] ? ("Image Array Out")
                (unwired) u64[] ? ("Histograms")
                w216 = bool ? ("Stop Measurement")
                n54 = call "HH_Stop.vi"("Device Index"=w217, "error in (no error)"=w219) -> ("error out"=w218:errorcluster)  [unwired: 12 in, 1 out]
              }
              frame #1 {
                # "Overflow Interv. Time (s)"
                # "No Error"
                n55 = call "PI Start WG.vi"("System no."=w244, "axis"=w233, "Generator"=T10 ?, "Init DDL"=T11 ?, "increment"=T11 ?, "error in"=w245, "saved data"=T12 ?) -> ("error out"=w246:errorcluster)  [unwired: 12 in]
                n56 = Initialize Array(i32 ?, i32 ?) -> (w224:i32[])
                n57 = while {
                  tunnel: w236 -> [w269]
                  tunnel: w243 -> [w285]
                  tunnel: w242 -> [w284]
                  shift-right: [w270] -> w248
                  shift-left: w246 -> [w286]
                  shift-right: [bool ? ("Reset")] -> _
                  shift-left: bool ? ("Reset") -> [w257]
                  tunnel: [w278] -> w241
                  tunnel: [w274] -> w240
                  tunnel: w239 -> [w276]
                  tunnel: [w275] -> w238
                  tunnel: [w253] -> w237
                  tunnel: [w252] -> w230
                  shift-right: [w266] -> w229
                  shift-left: w224 -> [w264]
                  tunnel: [w263] -> w228
                  tunnel: w223 -> [w260]
                  tunnel: w222 -> [_]
                  shift-right: [w251] -> w220
                  shift-left: w221 -> [w259]
                  i -> [w262]
                  stop <- w283 stop-if-true
                  n58 = call "HH_FIFORead.vi"("Device Index"=w269, "Buffer In"=w285, "Count"=w284, "error in (no error)"=w286) -> ("OK"=w279:bool, "Buffer Out"=w256:u32[], "Data Count"=w255:i32, "FiFo Overrun"=w278:bool, "error out"=w277:errorcluster)  [unwired: 7 in]
                  n59 = Unbundle(w277) -> ("status"=w282:bool)  [unwired: 2 out]
                  n60 = local write "Buffer Overrun"(w278) -> ()
                  n61 = call "HT3_Write.vi"("error in"=w277, "Data Count"=w255, "Data in"=w256, "refnum in"=w276) -> ("error out"=w271:errorcluster, "refnum out"=w275:refnum<file>)  [unwired: 6 in]
                  n62 = call "GetCountRates.vi"("error in (no error)"=w271, "DeviceIndex"=w269) -> ("error out"=w270:errorcluster, "CntRates"=w268:dbl[], "SyncRate"=w261:i32)  [unwired: 1 in]
                  n63 = local read "Stop Measurement"() -> (w273:bool)
                  n64 = local read "Global Stop"() -> (w272:bool)
                  n65 = Multiply(x=w260, y=w261) -> (x*y=w250:i32)
                  n66 = Compound Arithmetic op=OR(invert w279, w282, w272, w273) -> (w283:bool)
                  n67 = Insert Into Array(array=w268, index=i32 ?, new element=w261) -> (w265:dbl[])
                  n68 = call "HH_ToImage.vi"("Data In"=w256, "Reset"=w257, "Image Array In"=w259, "Data Count"=w255, "Pixel Time (Laser Pulses)"=w250) -> ("Image Array Out"=w251:i32[][], "Histograms"=→"Histogram":i32[][], "Total Oveflow Count"=w252:u64, "Num Records Total"=w253:i64, "Traces"=→"Trace":i32[][])  [unwired: 4 in, 2 out]
                  n69 = Or(x=w273, y=w272) -> (x .or. y?=w274:bool)
                  n70 = Add(x=w264, y=w265) -> (x+y=w266:dbl[])
                  n71 = Wait (ms)(milliseconds to wait=u32 ?) -> ()  [unwired: 1 out]
                  n72 = Increment(x=w262) -> (x+1=w263:i32)
                }
                "Image" <- w220
                n73 = call "HH_Stop.vi"("Device Index"=w236, "error in (no error)"=w248) -> ("error out"=w249:errorcluster)  [unwired: 12 in, 1 out]
                n74 = Divide(x=w229, y=w228) -> (x/y=w227:dbl[])
              }
            }
            n75 = flat-sequence {
              tunnel: w124 -> [w189]
              tunnel: [w178] -> w50
              tunnel: w121 -> [w191]
              tunnel: w120 -> [w180]
              tunnel: w51 -> [w188]
              tunnel: [w187] -> w48
              tunnel: w116 -> [w185]
              tunnel: w115 -> [w184]
              tunnel: w114 -> [w174]
              tunnel: w109 -> [w179]
              tunnel: w72 -> [w175]
              tunnel: w71 -> [w171]
              frame #0 {
                # "Count Rate (per s)"
                # "Finish after Aquire Image"
                n76 = Multiply(x=w175, y=w174) -> (x*y=w173:dbl)
                n77 = Or(x=w180, y=w191) -> (x .or. y?=w190:bool)
                n78 = case shown="False" w190 {
                  tunnel: w189 -> [w196 w206]
                  tunnel: w188 -> [w194 w207]
                  tunnel: [w193 w207] -> w187
                  tunnel: [w195 w205] -> w186
                  tunnel: [enum16{"timeover", "manual", "overflow"} ? ("Stop Reason") w210] -> w181
                  tunnel: w180 -> [w192 w208]
                  frame #0 {
                    # "Stop WaveGen\nif Aborted"
                    n79 = case shown="True" w192 {
                      tunnel: w196 -> [w198 w203]
                      tunnel: [w198 w202] -> w195
                      tunnel: w194 -> [w199 w201]
                      tunnel: [w199 w201] -> w193
                      frame #0 {
                      }
                      frame #1 {
                        n80 = call "PI Write GPIB.vi"("System no."=w201, "String to send"=string ?, "error in"=w203) -> ("error out"=w202:errorcluster)  [unwired: 16 in]
                      }
                    }
                  }
                  frame #1 {
                    n81 = Select(t=enum16{"timeover", "manual", "overflow"} ? ("Stop Reason"), s=w208, f=enum16{"timeover", "manual", "overflow"} ? ("Stop Reason")) -> (s? t:f=w210:enum16{"timeover", "manual", "overflow"})
                    n82 = call "PI Write GPIB.vi"("System no."=w207, "String to send"=string ?, "error in"=w206) -> ("error out"=w205:errorcluster)  [unwired: 16 in]
                  }
                }
                n83 = Multiply(x=w173, y=dbl ?) -> (x*y=w183:dbl)
                n84 = property on="Property Node" class="Bool"("BoolText.Text"=string ? ("Caption.Text"), "BoolText.TextColor"=u32 ? ("Boolean Text.Colors:FG Color")) -> ()  [unwired: 2 in, 2 out]
                n85 = To Long Integer(number=w183) -> (32bit integer=w182:i32)
                n86 = call "HT3_Finish.vi"("FileHeaderPos"=w179, "Rates"=w171, "Stop Reason"=w181, "error in"=w186, "Num Records"=w184, "Stop After (ms)"=w182, "refnum in"=w185) -> ("error out"=w178:errorcluster)  [unwired: 4 in]
              }
            }
            n87 = local read "X-Position"() -> (w41:dbl)
            n88 = local read "Y-Position"() -> (w40:dbl)
            n89 = local read "Z-Position"() -> (w39:dbl)
            n90 = Subtract(x=w42, y=w41) -> (x-y=w38:dbl)
            n91 = Subtract(x=w42, y=w40) -> (x-y=w37:dbl)
            n92 = Subtract(x=w42, y=w39) -> (x-y=w36:dbl)
            n93 = global read "GlobalConAxisPI.vi" "Conn. Axes"() -> (w47:string[])
            n94 = call "AOTF-Trigger_1.vi"("Channel"="Laser  Profile", "error in (no error)"=w80, "Triggered"=bool ?, "lp"=w74, "ap"=w75) -> ("error out"=w81:errorcluster)  [unwired: 2 in]
            n95 = Build Array(w38, w37, w36) -> (w46:dbl[])
            n96 = call "MOV.vi"("System no."=w48, "Axes to move"=w47, "Position values"=w46, "error in"=w50) -> ("error out"=w49:errorcluster)  [unwired: 15 in]
          }
          frame #2 {
            w323 = i32 ?
            w328 = i32 ?
            w356 = i32 ?
            w384 = i32 ? ("dimension size")
            n97 = Index Array(array=w355) -> (element=w422)  [unwired: 1 in]
            n98 = Unbundle By Name(w422) -> ("Dev"=w341)
            n99 = Equal?(x=w397, y=T3 ? ("Task")) -> (x = y?=w293:bool)
            n100 = local read "concatenated string"() -> (w348:string)
            n101 = And(x=w293, y="Autopoint-Autofocus Z") -> (x .and. y?=w385:bool)
            n102 = Or(x="Point Defocussed Cam", y="Auto Defocussed Cam") -> (x .or. y?=w310:bool)
            n103 = Select(t="Auto Measurement Time (ms)", s=w293, f="Measurement Time") -> (s? t:f=w294:i32)
            n104 = local read "X-Position"() -> (w403:dbl)
            n105 = local read "Y-Position"() -> (w402:dbl)
            n106 = local read "Z-Position"() -> (w338:dbl)
            n107 = Select(t=string ? ("Measurement Type"), s=w293, f=string ? ("Measurement Type")) -> (s? t:f=w347:string)
            n108 = case shown="True" w310 {
              tunnel: [w424 w429] -> w303
              tunnel: w304 -> [w424 w430]
              tunnel: w294 -> [_ w427]
              frame #0 {
              }
              frame #1 {
                n109 = global read "GlobalSetGetConfigureCamera.vi" "Exposure"() -> (w425:sgl)
                n110 = Greater?(x=w425, y=w427) -> (0:w428:bool)
                n111 = case shown="False" w428 {
                  tunnel: w427 -> [_ w432]
                  tunnel: [w431 w432] -> w426
                  tunnel: w425 -> [w431 _]
                  frame #0 {
                  }
                  frame #1 {
                  }
                }
                n112 = call "PrepCamera.vi"("mesTime"=w426, "error out 2"=w430) -> ("error out"=w429:errorcluster)  [unwired: 25 in]
              }
            }
            n113 = Select(t=T3 ? ("Task"), s=w293, f=T9 ? ("Do Measurement")) -> (s? t:f=w396:T3)
            n114 = local read "NxtAutMesPoint"() -> (w342:i32)
            n115 = Multiply(x=w294, y=i32 ?) -> (x*y=w295:i32)
            n116 = local read "Pattern"() -> (w343:dbl[][])
            n117 = Concatenate Strings(w348, w347) -> (w346:string)
            n118 = Bundle("X-Position"=w403, "Y-Position"=w402, "Z-Position"=w338) -> (w387:T24)  [unwired: 1 in]
            n119 = call "MTS_AutoPointCords.vi"("Is Auto Point"=w293, "Cords In"=w387, "Next Auto Measure Point"=w342, "Pattern"=w343) -> ("Cords"=w374:T24)  [unwired: 7 in]
            n120 = Unbundle By Name(w374) -> ("X-Position"=w314:dbl, "Y-Position"=w315:dbl, "Z-Position"=w324:dbl)
            n121 = Subtract(x=w328, y=w315) -> (x-y=w327:dbl)
            n122 = Subtract(x=w328, y=w314) -> (x-y=w326:dbl)
            n123 = Subtract(x=w328, y=w324) -> (x-y=w325:dbl)
            n124 = local read "PI SystemNumber"() -> (w336:i32)
            n125 = global read "GlobalConAxisPI.vi" "Conn. Axes"() -> (w330:string[])
            n126 = Build Array(w327, w326, w325) -> (w329:dbl[])
            n127 = local read "Last Image File No"() -> (w390:i32)
            n128 = call "MOV.vi"("System no."=w336, "Axes to move"=w330, "Position values"=w329, "No.of digits"=i16 ?, "error in"=w305) -> ("error out"=w318:errorcluster)  [unwired: 14 in]
            n129 = flat-sequence {
              tunnel: w318 -> [w433]
              tunnel: [w433] -> w317
              frame #0 {
                n130 = Wait (ms)(milliseconds to wait=u32 ?) -> ()  [unwired: 1 out]
              }
            }
            n131 = Select(t=T13 ? ("Measurement Type"), s=w293, f=T13 ? ("Measurement Type")) -> (s? t:f=w391:T13)
            n132 = Select(t=w390, s=w293, f=i32 ?) -> (s? t:f=w388:i32)
            n133 = local read "Workspace"() -> (w412:path)
            n134 = call "MTS_GenFileComment.vi"("Measurement Type"=w391, "Parent File No"=w388, "Info"=w352, "Upper Left"=w374, "error in"=w303) -> ("Comment"=w413:string, "error out"=w411:errorcluster)  [unwired: 7 in, 2 out]
            n135 = Not(x="Adjustment") -> (.not. x?=w350:bool)
            n136 = call "MTS_GetNextFileName.vi"("error in (no error)"=w411, "File Type"=string ?, "Measurement Type"=w346, "Workspace"=w412) -> ("error out"=w406:errorcluster, "Next File Name"=w405:path)  [unwired: 6 in]
            n137 = local read "CFD Settings"() -> (w381:T8)
            n138 = case shown="True" w350 {
              tunnel: w406 -> [w447 w455]
              tunnel: w405 -> [_ w454]
              tunnel: [w447 w453] -> w306
              tunnel: [path ? w448] -> w404
              tunnel: w391 -> [_ w450]
              tunnel: w388 -> [_ w452]
              tunnel: w386 -> [_ w449]
              frame #0 {
              }
              frame #1 {
                n139 = call "MTS_AddFileToWorkspace.vi"("File Name"=w454, "File Type"=T14 ?, "Measurement Type"=w450, "error in (no error)"=w455, "Parent"=w452, "Tree Refnum"=w449) -> ("File Name (dup)"=w448:path, "error out"=w453:errorcluster)  [unwired: 7 in, 1 out]
              }
            }
            n140 = call "POS?.vi"("System no."=w336, "Axes to query"=w330, "All axes?"=bool ?, "error in"=w317) -> ("Position"=w334:dbl[], "error out"=w337:errorcluster)  [unwired: 14 in]
            n141 = call "HH_Set.vi"("Device List"=w355, "CFD Settings"=w381, "error in (no error)"=w337) -> ("ht3 header out"=w401:T21, "Sync Rate"=w371:i32, "error out"=w399:errorcluster)  [unwired: 8 in, 2 out]
            n142 = Index Array(array=w334, index #1=i32 ? ("index"), index #2=i32 ? ("index"), index #3=i32 ? ("index")) -> (element #1=w322:dbl, element #2=w321:dbl, element #3=w320:dbl)
            n143 = Bundle By Name(cluster=w401, "AcquisitionTime (ms)"=w295) -> (w400:T21)
            n144 = Divide(x=i32 ? ("n"), y=w371) -> (x/y=w372:dbl)
            n145 = Subtract(x=w323, y=w322) -> (x-y=w292:dbl)
            n146 = Subtract(x=w323, y=w320) -> (x-y=w319:dbl)
            n147 = Subtract(x=w323, y=w321) -> (x-y=w291:dbl)
            n148 = property on="y-position" class="DigNum (strict)"("Value"=w292) -> ()  [unwired: 2 in, 2 out]
            n149 = property on="z-position" class="DigNum (strict)"("Value"=w319) -> ()  [unwired: 2 in, 2 out]
            n150 = case shown="True" w385 {
              tunnel: w399 -> [w456 w464]
              tunnel: [w456 w463] -> w398
              tunnel: w336 -> [_ w458]
              tunnel: w372 -> [_ w462]
              tunnel: w374 -> [_ w461]
              tunnel: w341 -> [_ w457]
              frame #0 {
              }
              frame #1 {
                # "Auto Z"
                n151 = call "MTS_AutoZPos.vi"("PH Dev"=w457, "OFlow Interv [s]"=w462, "PI System no."=w458, "error in"=w464, "Start Point"=w461) -> ("New Z"=w460:dbl, "Counts"=→"Counts":u32[], "error out"=w463:errorcluster)  [unwired: 8 in]
                n152 = local write "Z-Position"(w460) -> ()
              }
            }
            n153 = property on="x-position" class="DigNum (strict)"("Value"=w291) -> ()  [unwired: 2 in, 2 out]
            n154 = Initialize Array(u32 ?, w384) -> (w416:u32[])
            n155 = global read "ccdChipPixels.vi" "CCD Chip horizontal start"() -> (w301:i32)
            n156 = global read "ccdChipPixels.vi" "CCD Chip horizontal end"() -> (w302:i32)
            n157 = global read "ccdChipPixels.vi" "CCD Chip Vertical Start"() -> (w299:i32)
            n158 = global read "ccdChipPixels.vi" "CCD Chip Vertical end"() -> (w300:i32)
            n159 = Subtract(x=w302, y=w301) -> (x-y=w297:i32)
            n160 = Subtract(x=w300, y=w299) -> (x-y=w296:i32)
            n161 = flat-sequence {
              tunnel: w419 -> [w469]
              tunnel: w307 -> [w486]
              tunnel: [w467] -> w418
              tunnel: [w483] -> w354
              tunnel: w415 -> [w488]
              tunnel: w414 -> [w479]
              tunnel: w408 -> [w482]
              tunnel: w407 -> [w481]
              tunnel: w383 -> [w478]
              tunnel: w376 -> [w475]
              tunnel: w375 -> [w474]
              tunnel: w310 -> [w466]
              frame #0 {
                # "Finish after Measurement"
                n162 = case shown="False" w466 {
                  tunnel: w469 -> [w490 w495]
                  tunnel: [w490 w492] -> w468
                  frame #0 {
                  }
                  frame #1 {
                    n163 = call "SetShutter.vi"("type"=T16 ?, "mode"=T15 ?, "error in (no error)"=w495) -> ("error out"=w497:errorcluster)  [unwired: 11 in, 1 out]
                    n164 = call <vilib>:"Clear Errors.vi"("error in (no error)"=w497) -> ("error out"=w496:errorcluster)  [unwired: 6 in]
                    n165 = call "AbortAcquisition.vi"("error in (no error)"=w496) -> ("error out"=w491:errorcluster)  [unwired: 1 in, 1 out]
                    n166 = call <vilib>:"Clear Errors.vi"("error in (no error)"=w491) -> ("error out"=w492:errorcluster)  [unwired: 6 in]
                  }
                }
                n167 = Or(x=w479, y=w488) -> (x .or. y?=w487:bool)
                n168 = Index Array(array=w475, index=i32 ?) -> (element=w476:dbl)
                n169 = case shown="False" w487 {
                  tunnel: w486 -> [w499 w500]
                  tunnel: [w499 w500] -> w484
                  tunnel: [enum16{"timeover", "manual", "overflow"} ? ("Stop Reason") w503] -> w480
                  tunnel: w479 -> [_ w501]
                  frame #0 {
                  }
                  frame #1 {
                    n170 = Select(t=enum16{"timeover", "manual", "overflow"} ? ("Stop Reason"), s=w501, f=enum16{"timeover", "manual", "overflow"} ? ("Stop Reason")) -> (s? t:f=w503:enum16{"timeover", "manual", "overflow"})
                  }
                }
                n171 = Divide(x=w474, y=w476) -> (x/y=w473:dbl)
                n172 = Multiply(x=i32 ?, y=w473) -> (x*y=w471:dbl)
                n173 = To Long Integer(number=w471) -> (32bit integer=w470:i32)
                n174 = property on="Property Node" class="Bool"("BoolText.Text"=string ? ("Caption.Text"), "BoolText.TextColor"=u32 ? ("Boolean Text.Colors:FG Color")) -> ()  [unwired: 2 in, 2 out]
                n175 = call "HT3_Finish.vi"("FileHeaderPos"=w478, "Rates"=w475, "Stop Reason"=w480, "error in"=w484, "Num Records"=w481, "Stop After (ms)"=w470, "refnum in"=w482) -> ("error out"=w483:errorcluster)  [unwired: 4 in]
                n176 = Build Array(w469, w468) -> (w465:errorcluster[])
                n177 = call <vilib>:"Merge Errors.vi"("error array in"=w465) -> ("error out"=w467:errorcluster)  [unwired: 6 in]
              }
            }
            n178 = local read "Laser  Profile"() -> (w370:string)
            n179 = String To Byte Array(string=w370) -> (unsigned byte array=w368:u8[])
            n180 = Subtract(x=w368, y=i32 ?) -> (x-y=w363:i32[])
            n181 = String Length(string=w370) -> (length=w360:i32)
            n182 = Initialize Array(i32 ?, i32 ?, i32 ?) -> (w364:i32[][])
            n183 = Replace Array Subset(array=w364, new element=w363, index (col)=w356) -> (w362:i32[][])  [unwired: 1 in]
            n184 = Array Subset(array=w361, index=w356, length=w360) -> (w359:i32[])
            n185 = Replace Array Subset(array=w362, new element=w359, index (col)=i32 ?) -> (w358:i32[][])  [unwired: 1 in]
            n186 = call "HT3_Create.vi"("Laser"=w358, "Save pt3"=w350, "error in"=w398, "Comment"=w413, "ht3 Header in"=w400, "File Path"=w404) -> ("error out"=w339:errorcluster, "FileHeaderPos"=w383:T23, "refnum out"=w409:refnum<file>)  [unwired: 3 in]
            n187 = call "HH_Start.vi"("Device Index"=w341, "Acq. Time"=w295, "error in (no error)"=w339) -> ("error out"=w309:errorcluster)  [unwired: 11 in, 1 out]
            n188 = case shown="True" w310 {
              tunnel: [w435 w439] -> w289
              tunnel: w339 -> [w435 w438]
              tunnel: w293 -> [_ w437]
              tunnel: [_ w436] -> w298
              frame #0 {
              }
              frame #1 {
                n189 = control-ref of="NxtAutMesPoint"() -> (w444:refnum<vi>)
                n190 = control-ref of="Workspace"() -> (w445:refnum<vi>)
                n191 = control-ref of="y-position"() -> (w441:refnum<vi>)
                n192 = control-ref of="x-position"() -> (w442:refnum<vi>)
                n193 = control-ref of="z-position"() -> (w440:refnum<vi>)
                n194 = control-ref of="Pattern"() -> (w443:refnum<vi>)
                n195 = call "DefocussedImage.vi"("Path in"=w445, "reference"=w444, "Boolean"=w437, "reference 2"=w443, "reference 3"=w442, "error in (no error)"=w438, "reference 4"=w441, "reference 5"=w440) -> ("camout"=w436:i32[], "error out"=w439:errorcluster)  [unwired: 6 in]
              }
            }
            n196 = Unbundle By Name(w309) -> ("status"=w421:bool)
            n197 = Not(x=w421) -> (.not. x?=w420:bool)
            n198 = case shown="True" w420 {
              tunnel: [w511 w514] -> w308
              tunnel: w309 -> [w512 w523]
              tunnel: w306 -> [w513 w534]
              tunnel: [w513 w533] -> w419
              tunnel: w341 -> [w506 w522]
              tunnel: w416 -> [_ w530]
              tunnel: w384 -> [_ w529]
              tunnel: [w510 w528] -> w415
              tunnel: [w510 w527] -> w414
              tunnel: w409 -> [w509 w526]
              tunnel: [w509 w525] -> w408
              tunnel: [i64 ? ("Num Records Total") w524] -> w407
              tunnel: [dbl[] ? w519] -> w376
              tunnel: [i32 ? w518] -> w375
              frame #0 {
                w510 = bool ? ("Stop Measurement")
                n199 = call "HH_Stop.vi"("Device Index"=w506, "error in (no error)"=w512) -> ("error out"=w511:errorcluster)  [unwired: 12 in, 1 out]
              }
              frame #1 {
                # "Overflow Interv. Time (s)"
                # "No Error"
                n200 = Initialize Array(i32 ?, i32 ?) -> (w517:i32[])
                n201 = while {
                  tunnel: w522 -> [w543]
                  tunnel: w530 -> [w567]
                  tunnel: w529 -> [w566]
                  shift-right: [w544] -> w532
                  shift-left: w523 -> [w568]
                  shift-right: [w565] -> w533
                  shift-left: w534 -> [w565]
                  shift-right: [bool ? ("Reset")] -> _
                  shift-left: bool ? ("Reset") -> [w561]
                  tunnel: [w558] -> w528
                  tunnel: [w550] -> w527
                  tunnel: w526 -> [w554]
                  tunnel: [w553] -> w525
                  tunnel: [w552] -> w524
                  tunnel: [w551] -> w518
                  shift-right: [w538] -> w520
                  shift-left: w517 -> [w537]
                  tunnel: [w535] -> w521
                  i -> [w536]
                  stop <- w564 stop-if-true
                  n202 = call "HH_FIFORead.vi"("Device Index"=w543, "Buffer In"=w567, "Count"=w566, "error in (no error)"=w568) -> ("OK"=w559:bool, "Buffer Out"=w555:u32[], "Data Count"=w556:i32, "FiFo Overrun"=w558:bool, "error out"=w557:errorcluster)  [unwired: 7 in]
                  n203 = Wait (ms)(milliseconds to wait=u32 ?) -> ()  [unwired: 1 out]
                  n204 = Unbundle(w557) -> ("status"=w563:bool)  [unwired: 2 out]
                  n205 = local write "Buffer Overrun"(w558) -> ()
                  n206 = call "HT3_Write.vi"("error in"=w557, "Data Count"=w556, "Data in"=w555, "refnum in"=w554) -> ("error out"=w545:errorcluster, "refnum out"=w553:refnum<file>)  [unwired: 6 in]
                  n207 = call "HH_TraceAndHisto.vi"("Data In"=w555, "Reset"=w561, "Data Count"=w556) -> ("Histograms"=w547:i32[][], "Total Oveflow Count"=w551:u64, "Num Records Total"=w552:i64, "Traces"=w546:i32[][])  [unwired: 8 in, 1 out]
                  n208 = local read "Stop Measurement"() -> (w549:bool)
                  n209 = local read "Global Stop"() -> (w548:bool)
                  n210 = local write "Trace"(w546) -> ()
                  n211 = call "GetCountRates.vi"("error in (no error)"=w545, "DeviceIndex"=w543) -> ("error out"=w544:errorcluster, "CntRates"=w539:dbl[], "SyncRate"=w540:i32)  [unwired: 1 in]
                  n212 = Compound Arithmetic op=OR(invert w559, w563, w548, w549) -> (w564:bool)
                  n213 = local write "Histogram"(w547) -> ()
                  n214 = Insert Into Array(array=w539, index=i32 ?, new element=w540) -> (w541:dbl[])
                  n215 = Or(x=w549, y=w548) -> (x .or. y?=w550:bool)
                  n216 = Add(x=w537, y=w541) -> (x+y=w538:dbl[])
                  n217 = Increment(x=w536) -> (x+1=w535:i32)
                }
                n218 = Divide(x=w520, y=w521) -> (x/y=w519:dbl[])
                n219 = call "HH_Stop.vi"("Device Index"=w522, "error in (no error)"=w532) -> ("error out"=w514:errorcluster)  [unwired: 12 in, 1 out]
              }
            }
            n220 = Reshape Array(w298, w297, w296) -> (w290:i32[][])
            n221 = property on="Point" class="IntGraph (strict)"(error in=w289, "Value"=w290) -> (error out=w288:errorcluster)  [unwired: 1 in, 1 out]
            n222 = Build Array(w308, w288) -> (w287:errorcluster[])
            n223 = call <vilib>:"Merge Errors.vi"("error array in"=w287) -> ("error out"=w307:errorcluster)  [unwired: 6 in]
            n224 = call "AOTF-Trigger_1.vi"("Channel"=w370, "Pulse length"=w361, "Sync trigger ratio"=i32 ?, "error in (no error)"=w305, "Triggered"=bool ?) -> ("error out"=w379:errorcluster)  [unwired: 2 in]
            n225 = call "MOV.vi"("System no."=w336, "Axes to move"=w330, "Position values"=w329, "error in"=w354) -> ("error out"=w353:errorcluster)  [unwired: 15 in]
          }
          frame #3 {
            n226 = local read "Active pt3"() -> (w576:path)
            n227 = call "MTS_GetFileFromWS.vi"(".pt3 File Name"=w576) -> ("File Header"=w575:T25)  [unwired: 9 in, 1 out]
            n228 = Unbundle By Name(w575) -> ("Measurement Type"=w574:T26, "Pixels"=w571:i32[])
            n229 = control-ref of="WS File Tree"() -> (w577:refnum<vi>)
            n230 = Equal?(x=T13 ? ("Measurement Type"), y=w574) -> (x = y?=w572:bool)
            n231 = case shown="True" w572 {
              tunnel: w580 -> [w581 w604]
              tunnel: w576 -> [_ w603]
              tunnel: w576 -> [_ _]
              tunnel: [w581 w583] -> w569
              tunnel: w577 -> [_ _]
              tunnel: w571 -> [_ w588]
              frame #0 {
              }
              frame #1 {
                # "Image Intensity Array"
                # "Image Intensity Array"
                n232 = call "HT3_Open.vi"("error in"=w604, "File Path"=w603) -> ("error out"=w596:errorcluster, "Header"=w600:T27, "refnum out"=w602:refnum<file>)  [unwired: 3 in, 4 out]
                n233 = Unbundle By Name(w600) -> ()  [unwired: 15 out]
                n234 = Index Array(array=w588, index #2=i32 ? ("index")) -> (element #1=w585:i32, element #2=w586:i32)  [unwired: 1 in]
                n235 = Initialize Array(i32 ? ("element"), w585, w586) -> (w598:i32[][])
                n236 = Initialize Array(i32 ? ("element"), i32 ? ("dimension size"), w585, w586) -> (w591:i32[][][])
                n237 = while {
                  tunnel: w602 -> [w629]
                  shift-right: [bool ? ("Start From Top")] -> _
                  shift-left: bool ? ("Start From Top") -> [w623]
                  shift-right: [w622] -> w595
                  shift-left: w596 -> [w620]
                  tunnel: [w621] -> w594
                  tunnel: w598 -> [w619]
                  tunnel: [w618] -> w597
                  tunnel: [w619] -> _
                  stop <- w626 stop-if-true
                  n238 = call "HT3_Read.vi"("Start From Top"=w623, "error in"=w620, "Data count"=i32 ?, "refnum in"=w629) -> ("error out"=w622:errorcluster, "Data out"=w625:u32[], "refnum out"=w621:refnum<file>, "EOF?"=w626:bool)  [unwired: 4 in]
                  n239 = Array Size(array=w625) -> (size(s)=w624:i32)
                  n240 = call "HH_FileToImage_1.vi"("Data In"=w625, "Reset"=w623, "Data Count"=w624) -> ("Histograms"=w618:i32[][])  [unwired: 7 in, 5 out]
                }
                n241 = call "MTS_SelectTCSPCBinning.vi"("Histograms in"=w597) -> ("TCSPC Binning"=w590:i32[][])  [unwired: 1 in, 9 out]
                n242 = while {
                  tunnel: w594 -> [w617]
                  shift-right: [bool ? ("Start From Top")] -> _
                  shift-left: bool ? ("Start From Top") -> [w611]
                  shift-right: [w610] -> w582
                  shift-left: w595 -> [w606]
                  tunnel: [w609] -> w584
                  tunnel: w591 -> [w608]
                  tunnel: [w607] -> _
                  tunnel: w590 -> [w605]
                  stop <- w614 stop-if-true
                  n243 = call "HT3_Read.vi"("Start From Top"=w611, "error in"=w606, "Data count"=i32 ?, "refnum in"=w617) -> ("error out"=w610:errorcluster, "Data out"=w613:u32[], "refnum out"=w609:refnum<file>, "EOF?"=w614:bool)  [unwired: 4 out]
                  n244 = Array Size(array=w613) -> (size(s)=w612:i32)
                  n245 = call "HH_ToColorImage.vi"("Data In"=w613, "Reset"=w611, "Image Array In"=w608, "Data Count"=w612, "TCSPC Binning"=w605) -> ("Image Array Out"=w607:i32[][][])  [unwired: 2 in, 8 out]
                }
                n246 = Close File(refnum=w584, error in=w582) -> (error out=w583:errorcluster)  [unwired: 1 out]
              }
            }
          }
          frame #4 {
            # "dirty trick"
            n247 = local read "Active pt3"() -> (w656:path)
            n248 = call "MTS_GetFileFromWS.vi"(".pt3 File Name"=w656) -> ("File Header"=w655:T25)  [unwired: 9 in, 1 out]
            n249 = Unbundle By Name(w655) -> ("Measurement Type"=w654:T26, "Pixels"=w642:i32[], "Upper Left"=w651:T28, "Scan Axis"=w650:enum32{"x-y", "x-z", "y-z"})
            n250 = local read "Picture size 2"() -> (w637:dbl)
            n251 = local read "Picture size"() -> (w640:dbl)
            n252 = local read "Resolution"() -> (w638:dbl)
            n253 = local read "X-Position"() -> (w631:dbl)
            n254 = local read "Y-Position"() -> (w630:dbl)
            n255 = Divide(x=w640, y=w638) -> (x/y=w639:dbl)
            n256 = Divide(x=w637, y=w638) -> (x/y=w636:dbl)
            n257 = Equal?(x=T13 ? ("Measurement Type"), y=w654) -> (x = y?=w652:bool)
            n258 = call "MTS_ScannerXYZToImageXY.vi"("Axis"=w650, "Scanner XYZ"=w651) -> ("Image Y"=w633:dbl, "Image X"=w635:dbl)
            n259 = case shown="True" bool ? {
              tunnel: [w659 w662] -> w641
              tunnel: w642 -> [w659 _]
              tunnel: w639 -> [_ w666]
              tunnel: w636 -> [_ w665]
              tunnel: [w658 w661] -> w634
              tunnel: w635 -> [w658 _]
              tunnel: [w657 w660] -> w632
              tunnel: w633 -> [w657 _]
              tunnel: w631 -> [_ w661]
              tunnel: w630 -> [_ w660]
              frame #0 {
              }
              frame #1 {
                n260 = To Long Integer(number=w666) -> (32bit integer=w664:i32)
                n261 = To Long Integer(number=w665) -> (32bit integer=w663:i32)
                n262 = Build Array(w664, w663) -> (w662:i32[])
              }
            }
            n263 = Build Array(w640, w637) -> (w646:dbl[])
            n264 = case shown="True" w652 {
              tunnel: w649 -> [w667 w742]
              tunnel: w656 -> [_ _]
              tunnel: w656 -> [_ _]
              tunnel: [w667 w747] -> w647
              tunnel: w641 -> [_ w764]
              tunnel: w646 -> [_ w746]
              tunnel: w634 -> [_ w756]
              tunnel: w632 -> [_ w757]
              frame #0 {
              }
              frame #1 {
                w716 = T4 ? items=["Center of Mass X", "Center of Mass Y", "First Pixel X", "First Pixel Y", "Bounding Rect Left", "Bounding Rect Top", "Bounding Rect Right", "Bounding Rect Bottom", "Max Feret Diameter Start X", "Max Feret Diameter Start Y", "Max Feret Diameter End X", "Max Feret Diameter End Y", "Max Horiz. Segment Length Left", "Max Horiz. Segment Length Right", "Max Horiz. Segment Length Row", "-", "Bounding Rect Width", "Bounding Rect Height", "Bounding Rect Diagonal", "Perimeter", "Convex Hull Perimeter", "Holes' Perimeter", "Max Feret Diameter", "Equivalent Ellipse Major Axis", "Equivalent Ellipse Minor Axis", "Equivalent Ellipse Minor Axis (Feret)", "Equivalent Rect Long Side", "Equivalent Rect Short Side", "Equivalent Rect Diagonal", "Equivalent Rect Short Side (Feret)", "Average Horiz. Segment Length", "Average Vert. Segment Length", "Hydraulic Radius", "Waddel Disk Diameter", "-", "Area", "Holes' Area", "Particle & Holes' Area", "Convex Hull Area", "Image Area", "-", "Number of Holes", "Number of Horiz. Segments", "Number of Vert. Segments", "-", "Orientation", "Max Feret Diameter Orientation", "-", "% Area/Image Area", "% Area/(Particle & Holes' Area)", "Ratio of Equivalent Ellipse Axes", "Ratio of Equivalent Rect Sides", "-", "Elongation Factor", "Compactness Factor", "Heywood Circularity Factor", "Type Factor", "-", "Sum X", "Sum Y", "Sum XX", "Sum XY", "Sum YY", "Sum XXX", "Sum XXY", "Sum XYY", "Sum YYY", "-", "Moment of Inertia XX", "Moment of Inertia XY", "Moment of Inertia YY", "Moment of Inertia XXX", "Moment of Inertia XXY", "Moment of Inertia XYY", "Moment of Inertia YYY", "Norm. Moment of Inertia XX", "Norm. Moment of Inertia XY", "Norm. Moment of Inertia YY", "Norm. Moment of Inertia XXX", "Norm. Moment of Inertia XXY", "Norm. Moment of Inertia XYY", "Norm. Moment of Inertia YYY", "Hu Moment 1", "Hu Moment 2", "Hu Moment 3", "Hu Moment 4", "Hu Moment 5", "Hu Moment 6", "Hu Moment 7"] ("Measurement Parameter")
                w697 = bool ? ("Measurement Type")
                w721 = T4 ? items=["Center of Mass X", "Center of Mass Y", "First Pixel X", "First Pixel Y", "Bounding Rect Left", "Bounding Rect Top", "Bounding Rect Right", "Bounding Rect Bottom", "Max Feret Diameter Start X", "Max Feret Diameter Start Y", "Max Feret Diameter End X", "Max Feret Diameter End Y", "Max Horiz. Segment Length Left", "Max Horiz. Segment Length Right", "Max Horiz. Segment Length Row", "-", "Bounding Rect Width", "Bounding Rect Height", "Bounding Rect Diagonal", "Perimeter", "Convex Hull Perimeter", "Holes' Perimeter", "Max Feret Diameter", "Equivalent Ellipse Major Axis", "Equivalent Ellipse Minor Axis", "Equivalent Ellipse Minor Axis (Feret)", "Equivalent Rect Long Side", "Equivalent Rect Short Side", "Equivalent Rect Diagonal", "Equivalent Rect Short Side (Feret)", "Average Horiz. Segment Length", "Average Vert. Segment Length", "Hydraulic Radius", "Waddel Disk Diameter", "-", "Area", "Holes' Area", "Particle & Holes' Area", "Convex Hull Area", "Image Area", "-", "Number of Holes", "Number of Horiz. Segments", "Number of Vert. Segments", "-", "Orientation", "Max Feret Diameter Orientation", "-", "% Area/Image Area", "% Area/(Particle & Holes' Area)", "Ratio of Equivalent Ellipse Axes", "Ratio of Equivalent Rect Sides", "-", "Elongation Factor", "Compactness Factor", "Heywood Circularity Factor", "Type Factor", "-", "Sum X", "Sum Y", "Sum XX", "Sum XY", "Sum YY", "Sum XXX", "Sum XXY", "Sum XYY", "Sum YYY", "-", "Moment of Inertia XX", "Moment of Inertia XY", "Moment of Inertia YY", "Moment of Inertia XXX", "Moment of Inertia XXY", "Moment of Inertia XYY", "Moment of Inertia YYY", "Norm. Moment of Inertia XX", "Norm. Moment of Inertia XY", "Norm. Moment of Inertia YY", "Norm. Moment of Inertia XXX", "Norm. Moment of Inertia XXY", "Norm. Moment of Inertia XYY", "Norm. Moment of Inertia YYY", "Hu Moment 1", "Hu Moment 2", "Hu Moment 3", "Hu Moment 4", "Hu Moment 5", "Hu Moment 6", "Hu Moment 7"] ("Measurement Parameter")
                w736 = T29 ? items=["Grayscale (U8)", "Grayscale (I16)", "Grayscale (SGL)", "Complex (CSG)", "RGB (U32)", "HSL (U32)", "RGB (U64)", "Grayscale (U16)"] ("Image Type")
                w744 = T29 ? items=["Grayscale (U8)", "Grayscale (I16)", "Grayscale (SGL)", "Complex (CSG)", "RGB (U32)", "HSL (U32)", "RGB (U64)", "Grayscale (U16)"] ("Image Type")
                w763 = i32 ? ("index")
                # "Pixel Size [um]"
                n265 = Index Array(array=w746, index #2=w763) -> (element #1=w762:dbl, element #2=w759:dbl)  [unwired: 1 in]
                n266 = Index Array(array=w764, index #2=w763) -> (element #1=w761:i32, element #2=w760:i32)  [unwired: 1 in]
                n267 = Divide(x=w762, y=w761) -> (x/y=w672:dbl)
                n268 = Divide(x=w759, y=w760) -> (x/y=w758:dbl)
                n269 = Reciprocal(x=w672) -> (1/x=w673:dbl)
                n270 = Multiply(x=w673, y="Focuswidth") -> (x*y=w671:dbl)
                n271 = Random Number (0-1)() -> (number: 0 to 1=w741:dbl)
                n272 = Number To Decimal String(number=w741) -> (decimal integer string=w740:string)  [unwired: 1 in]
                n273 = Concatenate Strings(w740, string ? ("Image Name")) -> (w738:string)
                n274 = call "IMAQ Create"("Image Name"=w738, "Image Type"=w744, "error in (no error)"=w742) -> ("New Image"=w743:T2, "error out"=w731:errorcluster)  [unwired: 2 in]
                n275 = local read "Image"() -> (w675:i32[][])
                n276 = call "MTS_IntensityArrayToImage.vi"(0:"Image"=w743, 1:"Image"=w675, "error in (no error)"=w731, "Log Scale"=bool ?) -> ("Image Out"=w696:T2, "error out"=w688:errorcluster)  [unwired: 10 in]
                n277 = Random Number (0-1)() -> (number: 0 to 1=w735:dbl)
                n278 = Array To Cluster(array=T19 ? ("MesaurementSelection")) -> (cluster=w724:T30)
                n279 = Number To Decimal String(number=w735) -> (decimal integer string=w734:string)  [unwired: 1 in]
                n280 = Unbundle By Name(w724) -> ("MesaurementSelection[0]"=w722:T31, "MesaurementSelection[1]"=w717:T31, "MesaurementSelection[2]"=w712:T31, "MesaurementSelection[3]"=w703:T31)
                n281 = Concatenate Strings(w734, string ? ("Image Name")) -> (w732:string)
                n282 = call "IMAQ Create"("Image Name"=w732, "Image Type"=w736, "error in (no error)"=w688) -> ("New Image"=w730:T2, "error out"=w687:errorcluster)  [unwired: 2 in]
                n283 = Bundle By Name(cluster=w722, "Measurement Parameter"=w721, "Range Lower Value"="X Start 2", "Range Upper Value"="X End 2", "Range"="Exclude / Include X", "Measurement Type"=w697) -> (w711:T31)
                n284 = Bundle By Name(cluster=w717, "Measurement Parameter"=w716, "Range Lower Value"="Y Start 2", "Range Upper Value"="Y End 2", "Range"="Exclude / Include Y", "Measurement Type"=w697) -> (w710:T31)
                n285 = Bundle By Name(cluster=w712, "Measurement Parameter"="Measurement Parameter 1", "Range Lower Value"="Range Lower Value Par 1", "Range Upper Value"="Range Upper Value  Par 1", "Range"="Ex/In Par 1", "Measurement Type"=w697) -> (w709:T31)
                n286 = Bundle By Name(cluster=w703, "Measurement Parameter"="Measurement Parameter 2", "Range Lower Value"="Range Lower Value Par 2", "Range Upper Value"="Range Upper Value Par 2", "Range"="Ex/In Par 2", "Measurement Type"=w697) -> (w702:T31)
                n287 = Build Array(w711, w710, w709, w702) -> (w708:T19)
                n288 = call "MTS_IntensityArrayToImage.vi"(0:"Image"=w730, 1:"Image"=w675, "error in (no error)"=w687, "Log Scale"=bool ?) -> ("Image Out"=w681:T2, "error out"=w686:errorcluster)  [unwired: 10 in]
                n289 = case shown="0, Default" "Detection Modus" {
                  tunnel: "Remove Outliers" -> [_ w796]
                  tunnel: [w773 w787] -> w737
                  tunnel: w686 -> [w778 w795]
                  tunnel: [w771 w785] -> w728
                  tunnel: "Filter" -> [_ w794]
                  tunnel: w708 -> [_ w793]
                  tunnel: w696 -> [_ w788]
                  tunnel: path ? ("Template File Path (GeometricMatching)") -> [_ _]
                  tunnel: "Settings (GeometricMatching)" -> [_ _]
                  tunnel: T18 ? ("Rounding Mode Gaussian") -> [_ w792]
                  tunnel: T18 ? ("Rounding Mode Convolution") -> [_ w791]
                  tunnel: "Square/Hexa" -> [_ w790]
                  tunnel: "Connectivity 4/8" -> [_ w789]
                  tunnel: w681 -> [w775 w783]
                  tunnel: [w775 w780] -> w685
                  tunnel: [w777 w781] -> w683
                  tunnel: "Manual" -> [_ w779]
                  tunnel: w675 -> [w769 _]
                  tunnel: "Mode" -> [w768 _]
                  tunnel: w671 -> [w767 _]
                  tunnel: [w766 _] -> w669
                  tunnel: "NA" -> [w765 _]
                  frame #0 {
                    n290 = To Double Precision Float(number=w769) -> (double precision float=w770:dbl[][])
                    n291 = script code="addpath(path);\nswitch (mode)\ncase 0\nmaskGauss = GenGauss2D(focus);\n[err,bim,cim,sim,yc,xc,bc,cc,sc,len,imm]=FindPatternCP(image,maskGauss,[],[],[],1.5);\npattern=maskGauss;\ncase 1\nmaskRad=Radialpattern_gen('radial', focus,NA);\n[err,bim,cim,sim,yc,xc,bc,cc,sc,len,imm]=FindPatternCP(image,maskRad,[],[],[],1);\npattern=maskRad(:,:,15);\ncase 2\nmaskAzi=Radialpattern_gen('azimuthal', focus,NA);\n[err,bim,cim,sim,yc,xc,bc,cc,sc,len,imm]=FindPatternCP(image,maskAzi,[],[],[],1.5);\npattern=maskAzi(:,:,15);\nend\nxc=xc-1;\nyc=yc-1;"("??"=w778, "path"=string ?, "image"=w770, "mode"=w768, "focus"=w767, "NA"=w765) -> ("??"=w777:errorcluster, "pattern"=w766:dbl[][], "xc"=w774:dbl[], "yc"=w772:dbl[])
                    n292 = Build Array(w774, w772) -> (w773:dbl[][])
                    n293 = Array Size(array=w772) -> (size(s)=w771:i32)
                  }
                  frame #1 {
                    n294 = call "SingleMoleFinderEasy.vi"("Image Src"=w788, "Number of Erosion"=w796, "HolesBorder"=w794, "Selection Values"=w793, "Rounding Mode Gaussian"=w792, "error in"=w795, "Rounding Mode Convolution"=w791, "Square/Hexa (Square)"=w790, "Connectivity 4/8 (8)"=w789) -> ("Number of Particles"=w784:i32, "Particle Measurements (Pixels)"=w786:dbl[][], "error out"=w782:errorcluster)  [unwired: 15 in, 1 out]
                    n295 = case shown="True" w779 {
                      tunnel: w782 -> [w800 w808]
                      tunnel: [w800 w807] -> w781
                      tunnel: [w797 w806] -> w780
                      tunnel: [w798 w805] -> w787
                      tunnel: w786 -> [w798 w802]
                      tunnel: [w799 w804] -> w785
                      tunnel: w784 -> [w799 w803]
                      tunnel: w783 -> [w797 w801]
                      frame #0 {
                      }
                      frame #1 {
                        n296 = while {
                          tunnel: w808 -> [w823]
                          tunnel: [w822] -> w807
                          tunnel: w801 -> [w821]
                          tunnel: [w820] -> w806
                          shift-right: [w813] -> w805
                          shift-left: w802 -> [w812]
                          tunnel: [w811] -> w804
                          tunnel: w803 -> [w810]
                          i -> [w817]
                          stop <- w819 stop-if-true
                          n297 = call "IMAQ Select Point"("Window Number (0...15)"=i32 ?, "error in (no error)"=w823, "Image In"=w821) -> ("error out"=w822:errorcluster, "Cancelled"=w819:bool, "Point"=w818:T32, "Image Out (duplicate)"=w820:T2)  [unwired: 5 in]
                          n298 = Unbundle(w818) -> ("X"=w816:sgl, "Y"=w815:sgl)
                          n299 = Build Array(w816, w815) -> (w814:sgl[])
                          n300 = Add(x=w810, y=w817) -> (x+y=w811:i32)
                          n301 = Insert Into Array(array=w812, index (row)=w811, new element=w814) -> (w813:dbl[][])  [unwired: 1 in]
                        }
                      }
                    }
                  }
                }
                "Number of Particles" <- w728
                "Image 2" <- w669
                n302 = Index Array(array=w737, index (col) #1=i32 ? ("index (row)"), index (col) #2=i32 ? ("index (col)")) -> (element #1=w680:dbl[], element #2=w678:dbl[])  [unwired: 2 in]
                n303 = Multiply(x=w672, y=w680) -> (x*y=w755:dbl[])
                n304 = Multiply(x=w678, y=w758) -> (x*y=w754:dbl[])
                n305 = To Word Integer(number=w680) -> (16bit integer=w679:i16[])
                n306 = To Word Integer(number=w678) -> (16bit integer=w677:i16[])
                n307 = Add(x=w756, y=w755) -> (x+y=w750:dbl[])
                n308 = Add(x=w754, y=w757) -> (x+y=w749:dbl[])
                n309 = for {
                  N: w728 -> [_]
                  shift-right: [w830] -> w684
                  shift-left: w685 -> [w831]
                  tunnel: w679 -> [w829] mode=indexing
                  tunnel: w677 -> [w828] mode=indexing
                  shift-right: [w832] -> w682
                  shift-left: w683 -> [w833]
                  tunnel: u32 ? -> [w827]
                  tunnel: dbl ? ("x") -> [w826]
                  n310 = call "MTS_DrawCrossIMAQIamge.vi"("Image"=w831, "Size"=w826, "Color"=w827, "X"=w829, "Y"=w828, "error in (no error)"=w833) -> ("Image Out"=w830:T2, "error out"=w832:errorcluster)  [unwired: 8 in]
                }
                "AM image" <- w684
                n311 = Build Array(w750, w749, w679, w677) -> (→"Pattern":dbl[][])
                n312 = flat-sequence {
                  tunnel: w682 -> [w825]
                  tunnel: [w825] -> w747
                  frame #0 {
                    n313 = local write "Tab Control"(T1 ? ("Tab Control")) -> ()
                  }
                }
                n314 = global write "patternImg.vi" "New Image"(w684) -> ()
              }
            }
          }
          frame #5 {
            # "Init"
            n315 = local read "Pattern"() -> (w844:dbl[][])
            n316 = Index Array(array=w844, index (row) #1=i32 ? ("index (row)"), index (row) #2=i32 ? ("index (col)")) -> (element #1=w841:dbl[], element #2=→"subarray":dbl[])  [unwired: 2 in]
            n317 = local read "NxtAutMesPoint"() -> (w852:i32)
            n318 = Array Size(array=w841) -> (size(s)=w840:i32)
            n319 = Less Than 0?(x=w852) -> (x < 0?=w855:bool)
            n320 = case shown="False" w855 {
              tunnel: w849 -> [w876 w880]
              tunnel: [w876 w879] -> w853
              tunnel: [w875 w877] -> w851
              tunnel: w840 -> [_ w877]
              frame #0 {
                n321 = local read "Auto Measure Points"() -> (w875:i32)
              }
              frame #1 {
                n322 = Number To Decimal String(number=w877) -> (decimal integer string=w882:string)  [unwired: 1 in]
                n323 = Concatenate Strings(string ? ("Caption.Text"), w882) -> (w881:string)
                n324 = property on="Auto Meas Progress" class="Slide (strict)"(error in=w880, "Scale.Minimum"=dbl ? ("Scale.Range:Minimum"), "Scale.Maximum"=w877, "Value"=i32 ? ("Auto Meas Progress"), "Caption.Text"=w881) -> (error out=w879:errorcluster)  [unwired: 1 in, 1 out]
                "Auto Measure Points" <- w877
              }
            }
            n325 = Increment(x=w852) -> (x+1=w835:i32)
            "NxtAutMesPoint" <- w835
            n326 = Greater Or Equal?(x=w835, y=w851) -> (x >= y?=w854:bool)
            n327 = Increment(x=w835) -> (x+1=w850:i32)
            n328 = Index Array(array=w844, index (row) #1=i32 ? ("index (row)"), index (col) #1=w835, index (row) #2=i32 ? ("index (col)"), index (col) #2=w835) -> (element #1=w843:dbl, element #2=w842:dbl)
            n329 = case shown="False" w854 {
              tunnel: w853 -> [w866 w874]
              tunnel: [w872 w874] -> w847
              tunnel: [T17 ? ("Do Measurement") T17 ? ("Do Measurement")] -> w846
              tunnel: w850 -> [w867 _]
              tunnel: w843 -> [w864 _]
              tunnel: w842 -> [w863 _]
              tunnel: w851 -> [w860 _]
              frame #0 {
                # "Prpare For Next Point"
                # "1 loc max  2 undef 0 saddle -1 local min"
                n330 = global read "patternImg.vi" "New Image"() -> (w856:T2)
                n331 = Number To Decimal String(number=w867) -> (decimal integer string=w869:string)  [unwired: 1 in]
                n332 = Number To Decimal String(number=w860) -> (decimal integer string=w861:string)  [unwired: 1 in]
                n333 = Concatenate Strings(string ? ("Caption.Text"), w869, string ? ("Caption.Text"), w861) -> (w868:string)
                n334 = call "MTS_DrawCrossIMAQIamge.vi"("Image"=w856, "Size"=dbl ? ("x"), "Color"=u32 ?, "X"=w864, "Y"=w863, "error in (no error)"=w866) -> ("Image Out"=w857:T2, "error out"=w865:errorcluster)  [unwired: 8 in]
                n335 = property on="Auto Meas Progress" class="Slide (strict)"(error in=w865, "Value"=w867, "Caption.Text"=w868) -> (error out=w872:errorcluster)  [unwired: 1 in, 1 out]
                n336 = local write "AM image"(w857) -> ()
              }
              frame #1 {
                # "No More Points"
              }
            }
          }
        }
        n337 = local write "Buffer Overrun"(w22) -> ()
      }
      frame #1 {
      }
    }
    n338 = Unbundle(w7) -> ("status"=w6:bool)  [unwired: 2 out]
    n339 = flat-sequence {
      tunnel: w10 -> [w900]
      tunnel: [w900] -> w9
      tunnel: w5 -> [w897]
      frame #0 {
        n340 = local write "Task"(w897) -> ()
        n341 = Equal?(x=w897, y=T9 ? ("Do Measurement")) -> (x = y?=w898:bool)
        n342 = Not(x=w898) -> (.not. x?=w899:bool)
        n343 = local write "Running"(w899) -> ()
      }
    }
    n344 = local read "Global Stop"() -> (w13:bool)
    n345 = Compound Arithmetic op=OR(w6, w11, w13) -> (w12:bool)
  }
